vi "Collision Detection top level.vi"(0 "Model rotation (degrees)":sgl, 1 "Model rotation axis (unit vector)":sgl[](array[numeric])=[0.0, 0.0, 1.0], 2 "Traverse Active Parts":cluster{"X":bool, "XY":bool, "XYZ":bool}, 3 "Model rotation axis coordinates (absolute, mm)":sgl[](array[numeric])=[0.0, 0.0, 0.0], 4 "Collision mode":T1=enum."Traverse - All", 5 "Get minimum separation within look-out sphere":bool, 6 "Traverse position (absolute, mm)":sgl[](array[numeric])=[0.0, 0.0, 0.0], 7 "3D graphics output":bool, 9 "Visualisation only (no collision detection)":bool, 10 "Traverse name":string="EnFlo_Trav1", 11 "Extrusion mode":bool, 12 "Rig geometry directory path":path=path "C:/EnFlo_Data_Local/Preferences/Rig_Setups/EnFlo_Tunnel/All_Users/Collision_detection", 13 "Traverse extruded position":sgl[](array[numeric])=[0.0, 0.0, 0.0]) -> (14 "Collision":bool, 15 "Collision point(s)":sgl[][](array[numeric]), 16 "Traverse collision part":cluster{"X":bool, "XY":bool, "XYZ":bool}, 17 "Minimum separation":sgl, 18 "Minimum separation vector (from trav.)":sgl[](array[numeric]), 19 "Error out":errorcluster)   [LabVIEW 2020]
uses:
  Collision Mode.ctl
  Typedefs/Triangle.ctl
  <vilib>/Utility/miscctls.llb/LVRGBAColorTypeDef.ctl
  Convex Hull/Subroutines/Coincident points test.vi
  Subroutines/Cross product 3D.vi
  Subroutines/Unit vector.vi
  Query Octree with triangle.vi
  Tri-Tri intersection test.vi
  Subroutines/Triangle-NodeBox containment test.vi
  Subroutines/Edge-Tri intersection test.vi
  Subroutines/TriVert-in-Box test.vi
  Subroutines/BoxEdges-Tri intersection test.vi
  Subroutines/TriEdges-Box intersection test.vi
  Subroutines/Point-in-Tri test.vi
  Subroutines/Edge-Plane intersection test.vi
  Subroutines/Point-in-Box test (axis-aligned).vi
  Subroutines/Edge-Quad intersection test.vi
  Subroutines/Point-in-Quad test (axis-aligned).vi
  Collision Detection global.vi
  Globals/Trav_pos_global.vi
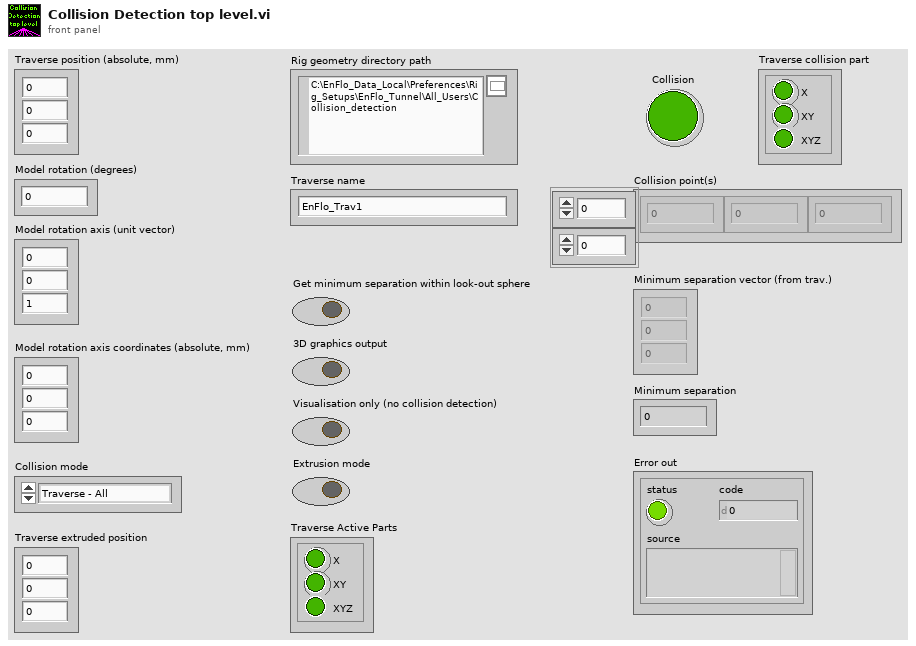
[diagram p1: front panel]
types:
  T1 = typedef "Collision Mode.ctl" = enum16{"Traverse - Tunnel", "Traverse - Model", "Traverse - Fixed objects", "Traverse - Traverse", "Traverse - All"}
  T2 = cluster{"Red":sgl, "Green":sgl, "Blue":sgl, "Alpha":sgl}
  T3 = typedef "LVRGBAColorTypeDef.ctl" = cluster{"Red":sgl, "Green":sgl, "Blue":sgl, "Alpha":sgl}
  T4 = typedef "TreeNodeBox.ctl" = cluster{"Face 0":T5, "Face 1":T5, "Face 2":T5, "Face 3":T5, "Face 4":T5, "Face 5":T5, "Level":i32, "Pmax":sgl[], "Pmin":sgl[], "Parent":i32, "Child 1":i32, "Child 2":i32, "Child 3":i32, "Child 4":i32, "Child 5":i32, "Child 6":i32, "Child 7":i32, "Child 8":i32, "Triangles":i32[], "is leaf node":bool}
  T5 = typedef "Quad.ctl" = cluster{"V0":sgl[], "V1":sgl[], "V2":sgl[], "V3":sgl[], "E0":sgl[], "E1":sgl[], "E2":sgl[], "E3":sgl[], "n^":sgl[], "Plane":T6}
  T6 = typedef "Quadplane enum.ctl" = enum8{"XY", "XZ", "YZ", "-XY", "-XZ", "-YZ"}
  T7 = typedef "Triangle.ctl" = cluster{"V0":sgl[], "V1":sgl[], "V2":sgl[], "E0":sgl[], "E1":sgl[], "E2":sgl[], "n^":sgl[], "nE0^":sgl[], "nE1^":sgl[], "nE2^":sgl[]}
  T8 = typedef "Sphere.ctl" = cluster{"Centre":sgl[], "Radius":sgl}
  T9 = typedef "Triangle, indexed.ctl" = cluster{"V0":sgl[], "V1":sgl[], "V2":sgl[], "n^":sgl[], "i0":i32, "i1":i32, "i2":i32}
  T10 = enum16{"Inherit Value", "Points", "Wireframe", "Polygons"}
  T11 = typedef "LV3DPointTypeDef.ctl" = cluster{"X":sgl, "Y":sgl, "Z":sgl}
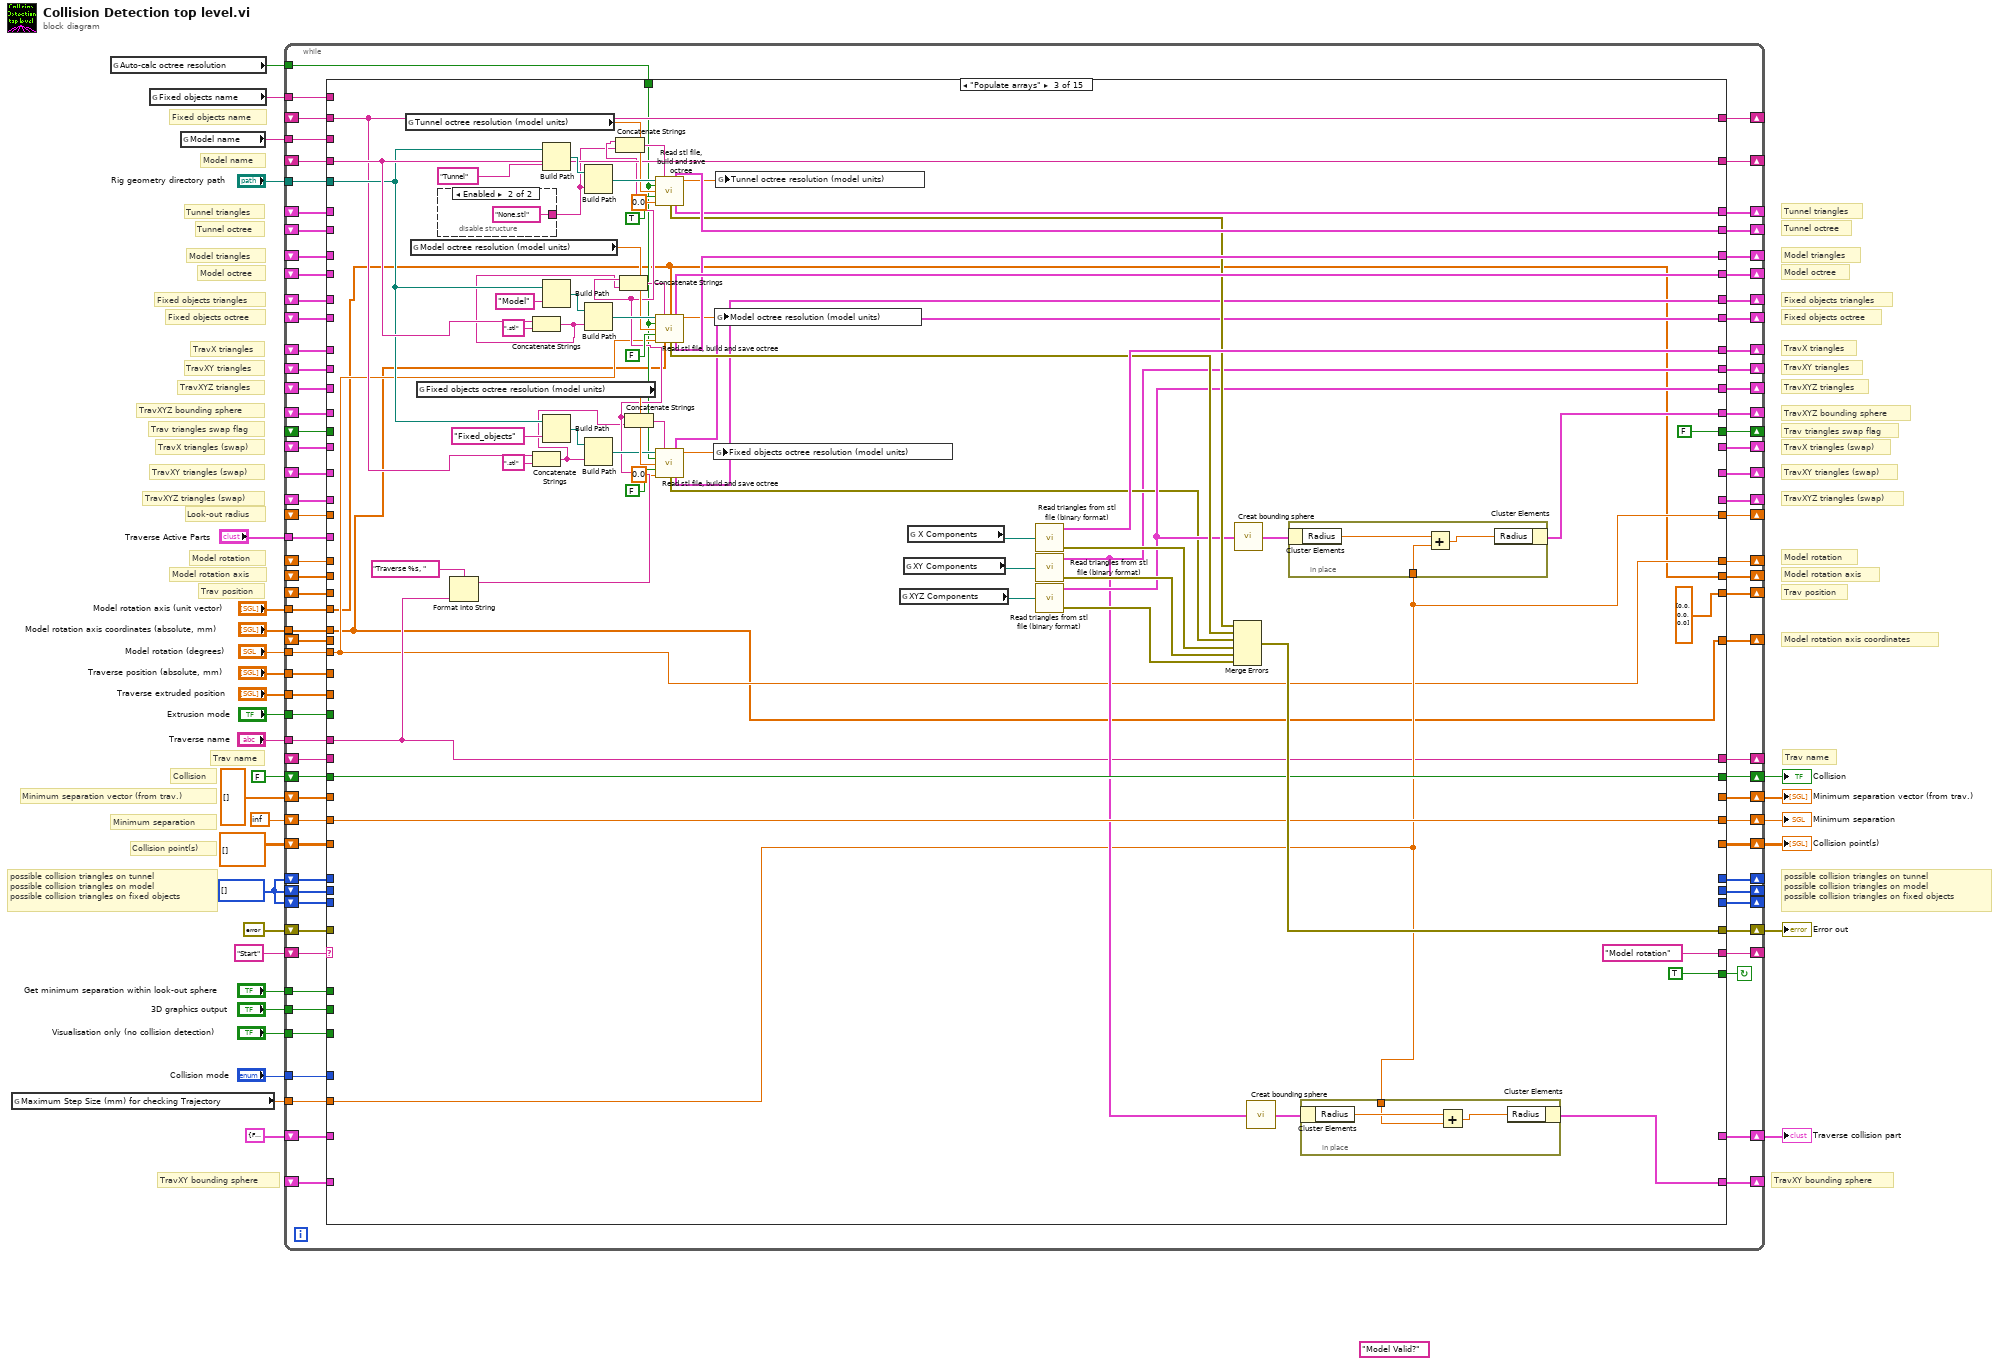
[diagram p0: block diagram]
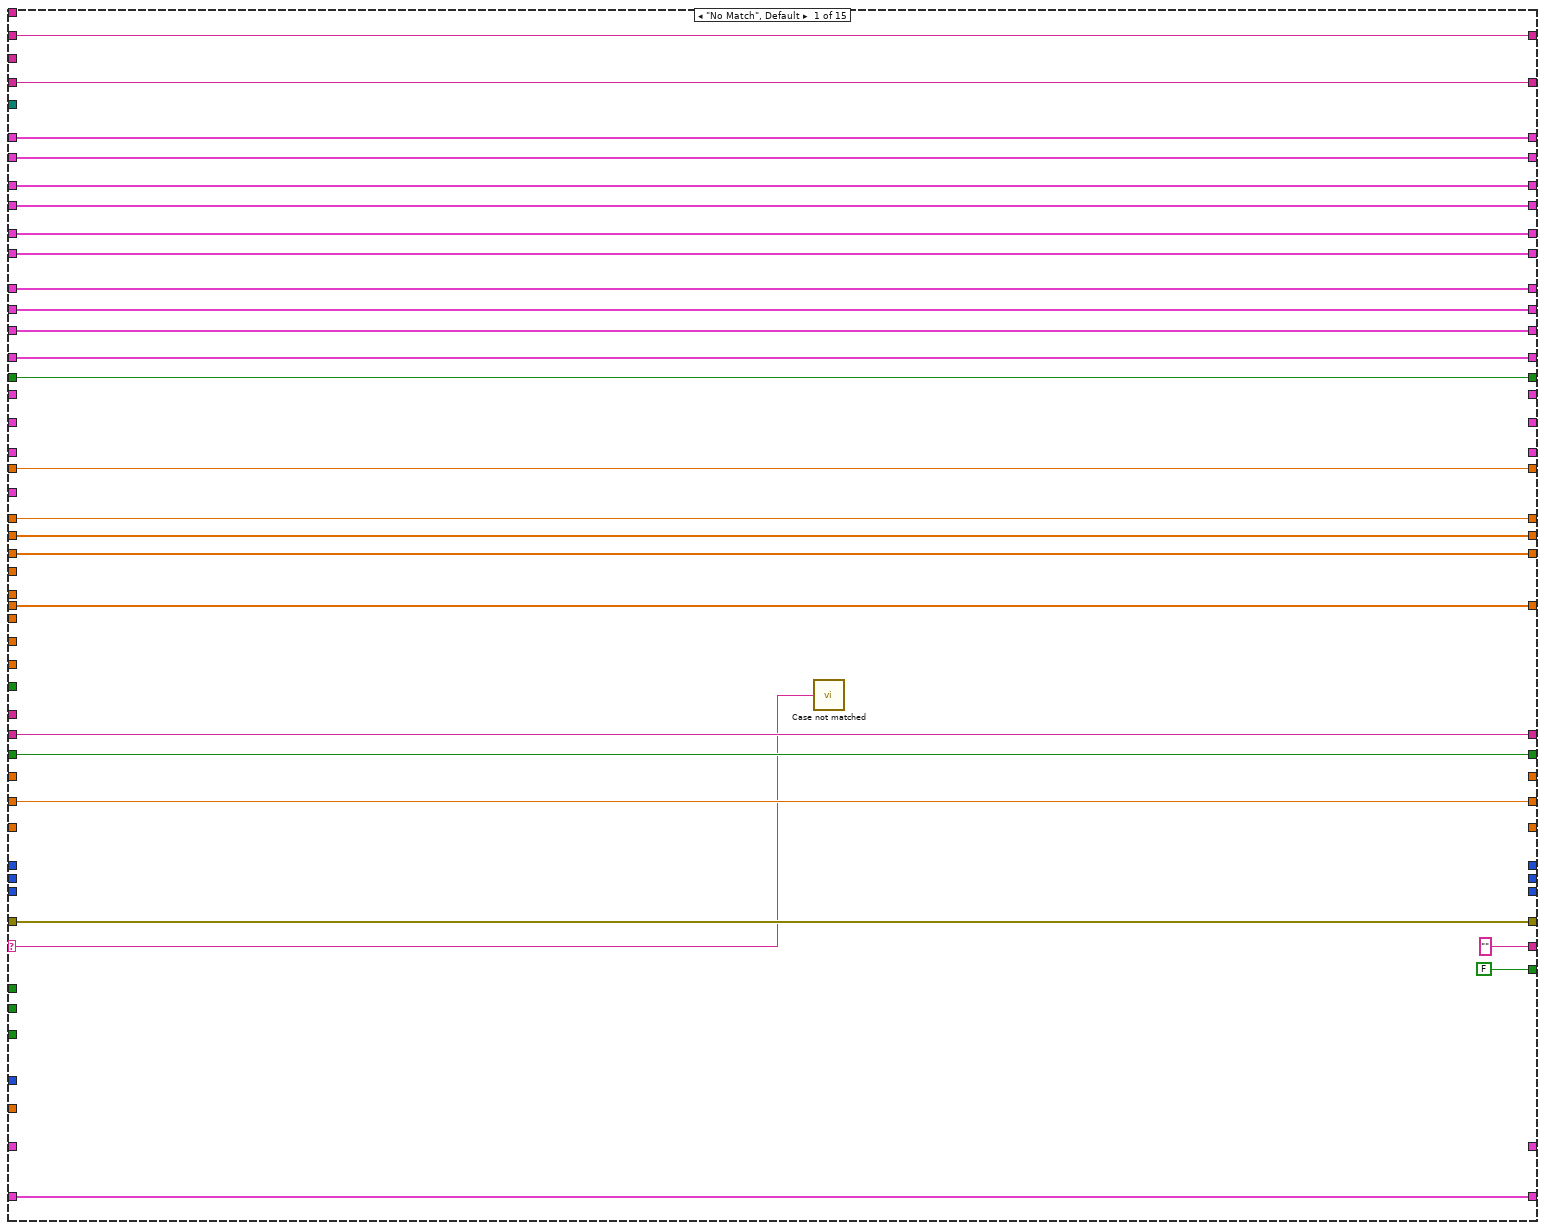
[diagram p2: hidden frame]
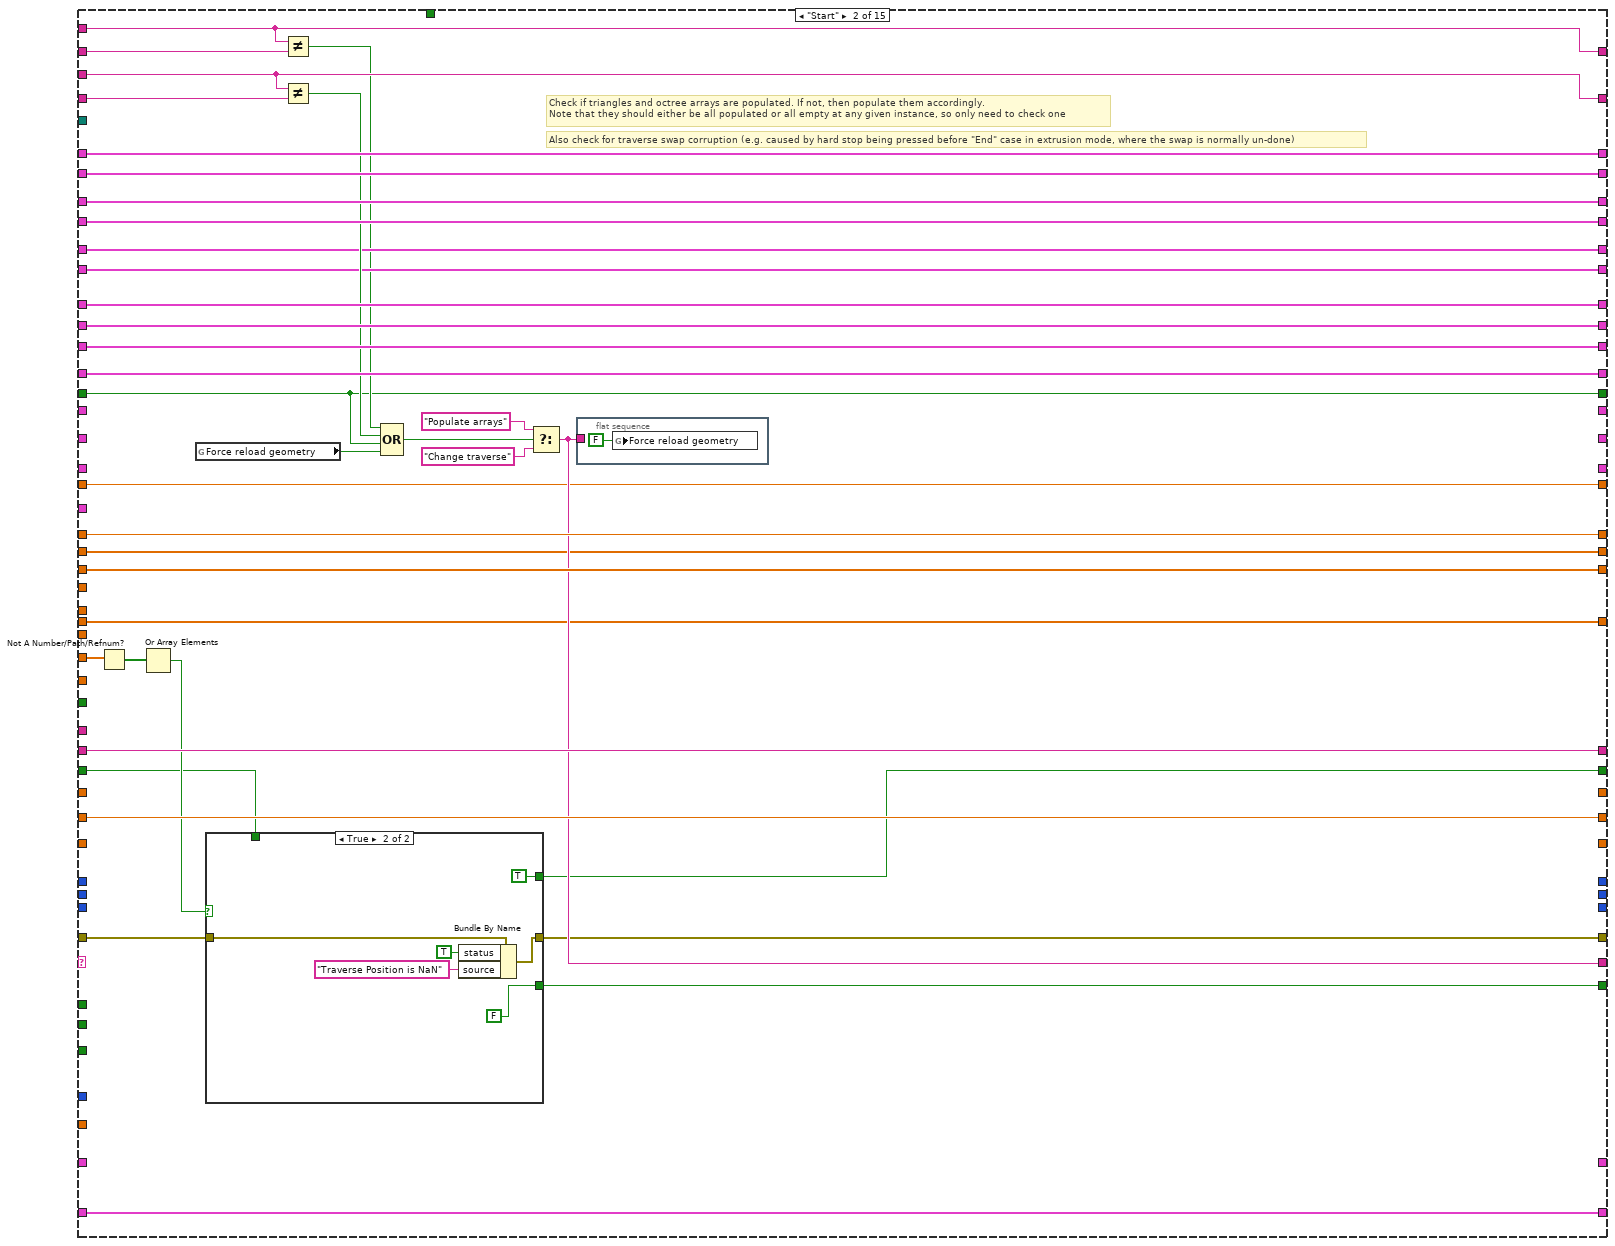
[diagram p3: hidden frame]
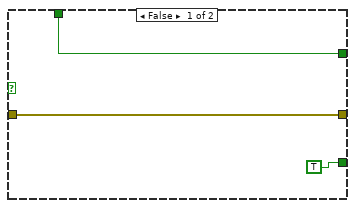
[diagram p4: hidden frame]
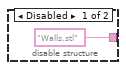
[diagram p5: hidden frame]
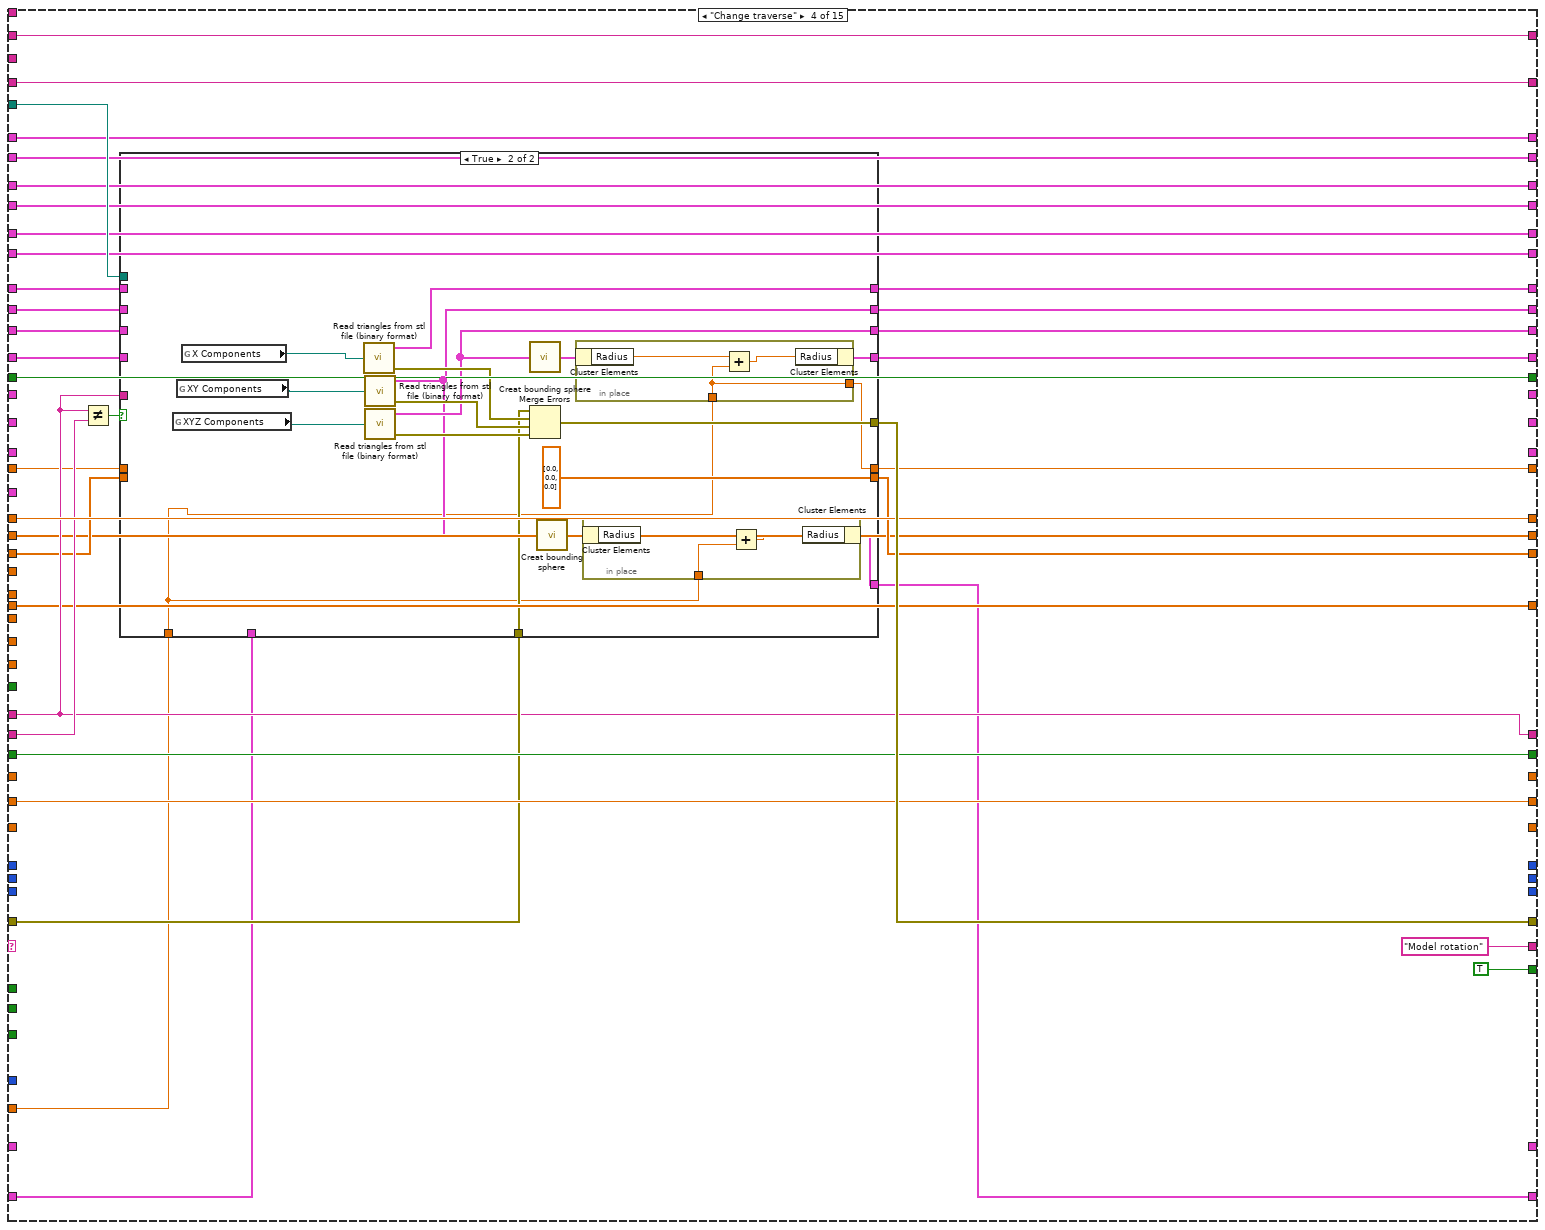
[diagram p6: hidden frame]
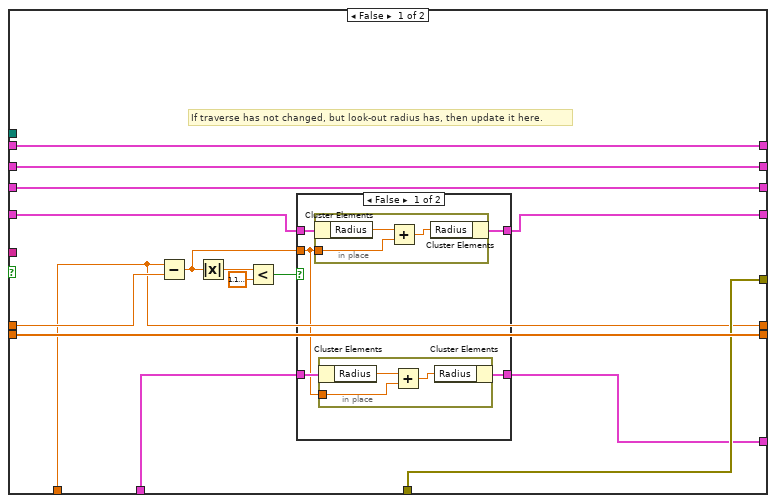
[diagram p7: hidden frame]
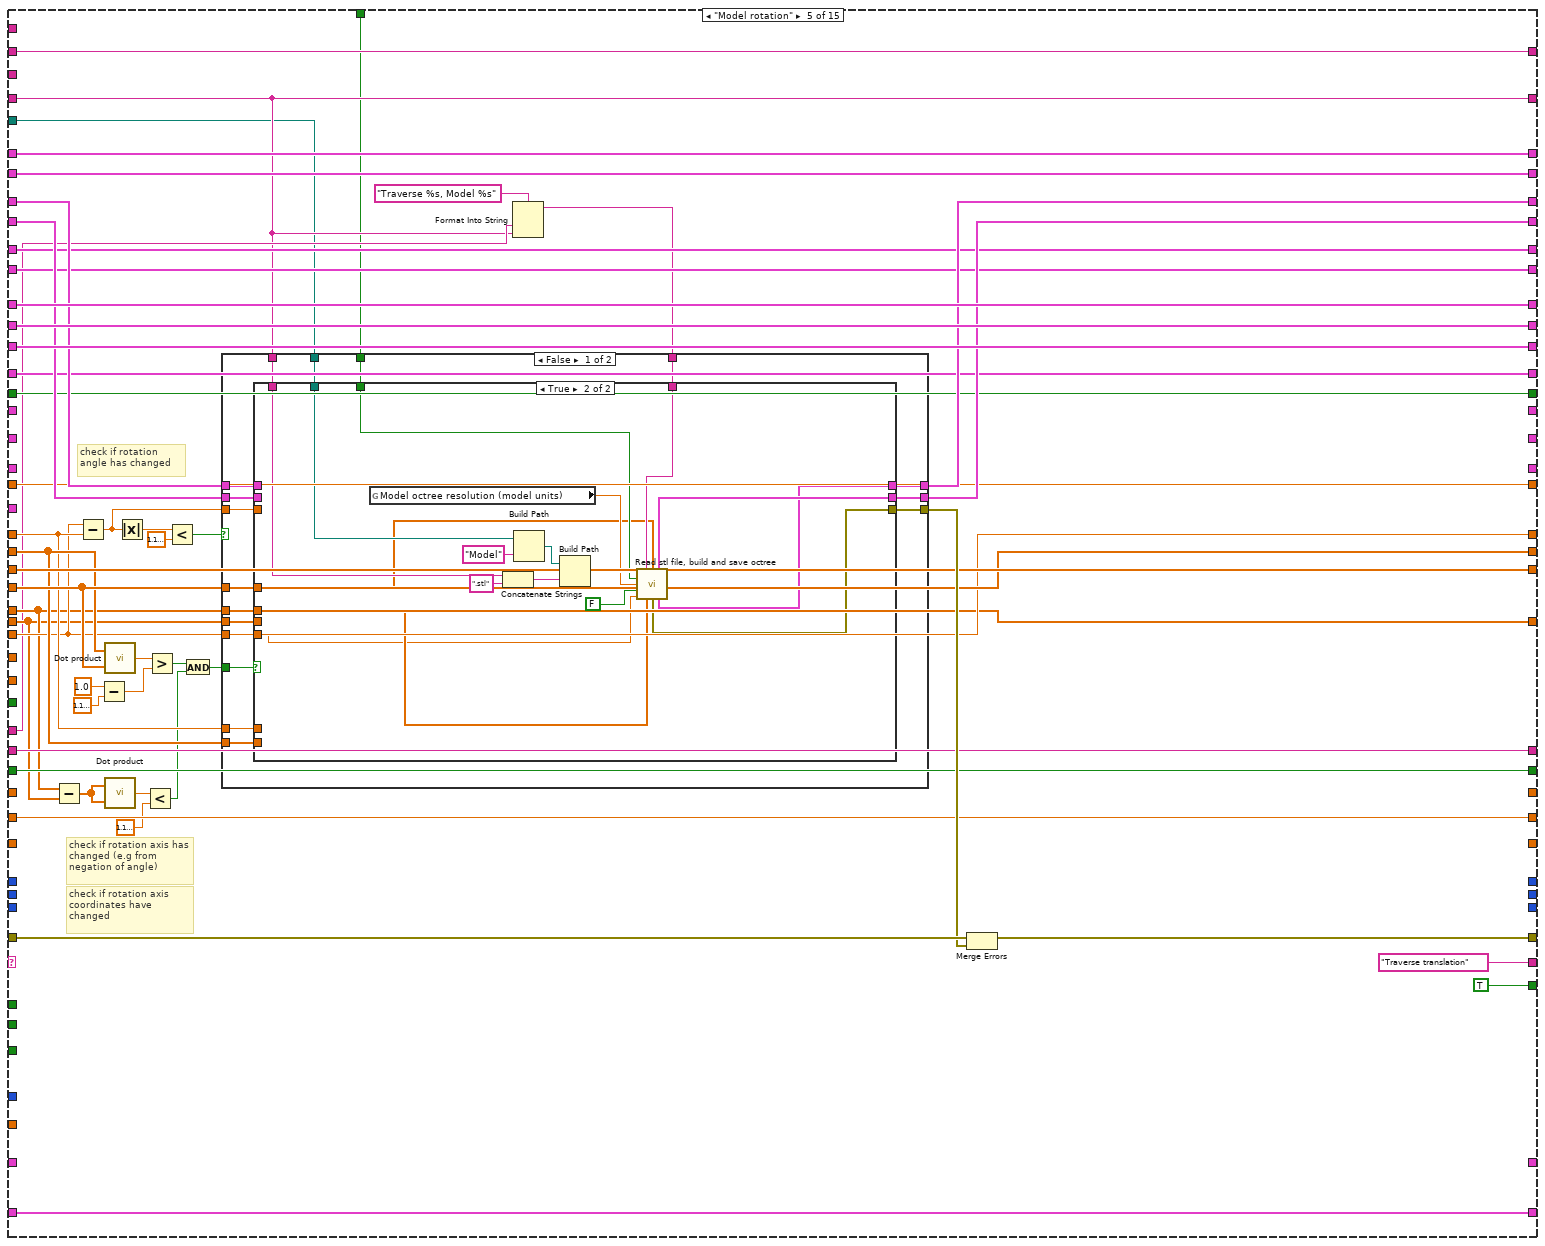
[diagram p9: hidden frame]
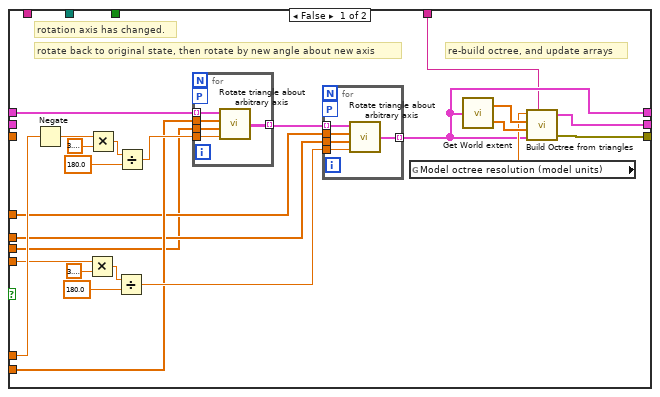
[diagram p10: hidden frame]
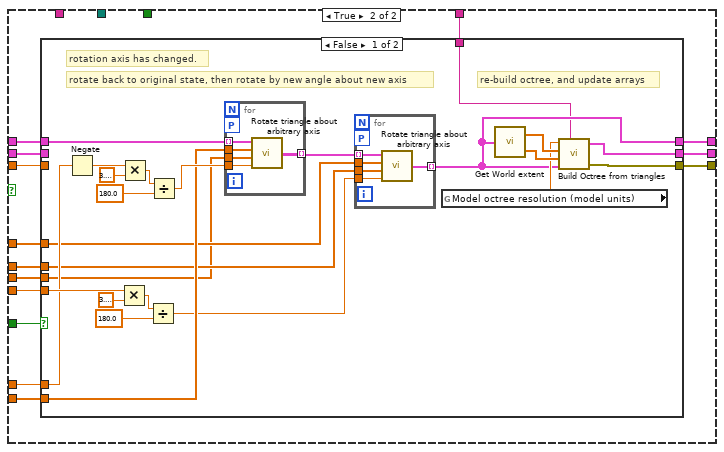
[diagram p11: hidden frame]
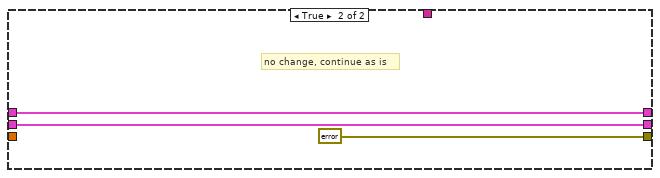
[diagram p12: hidden frame]
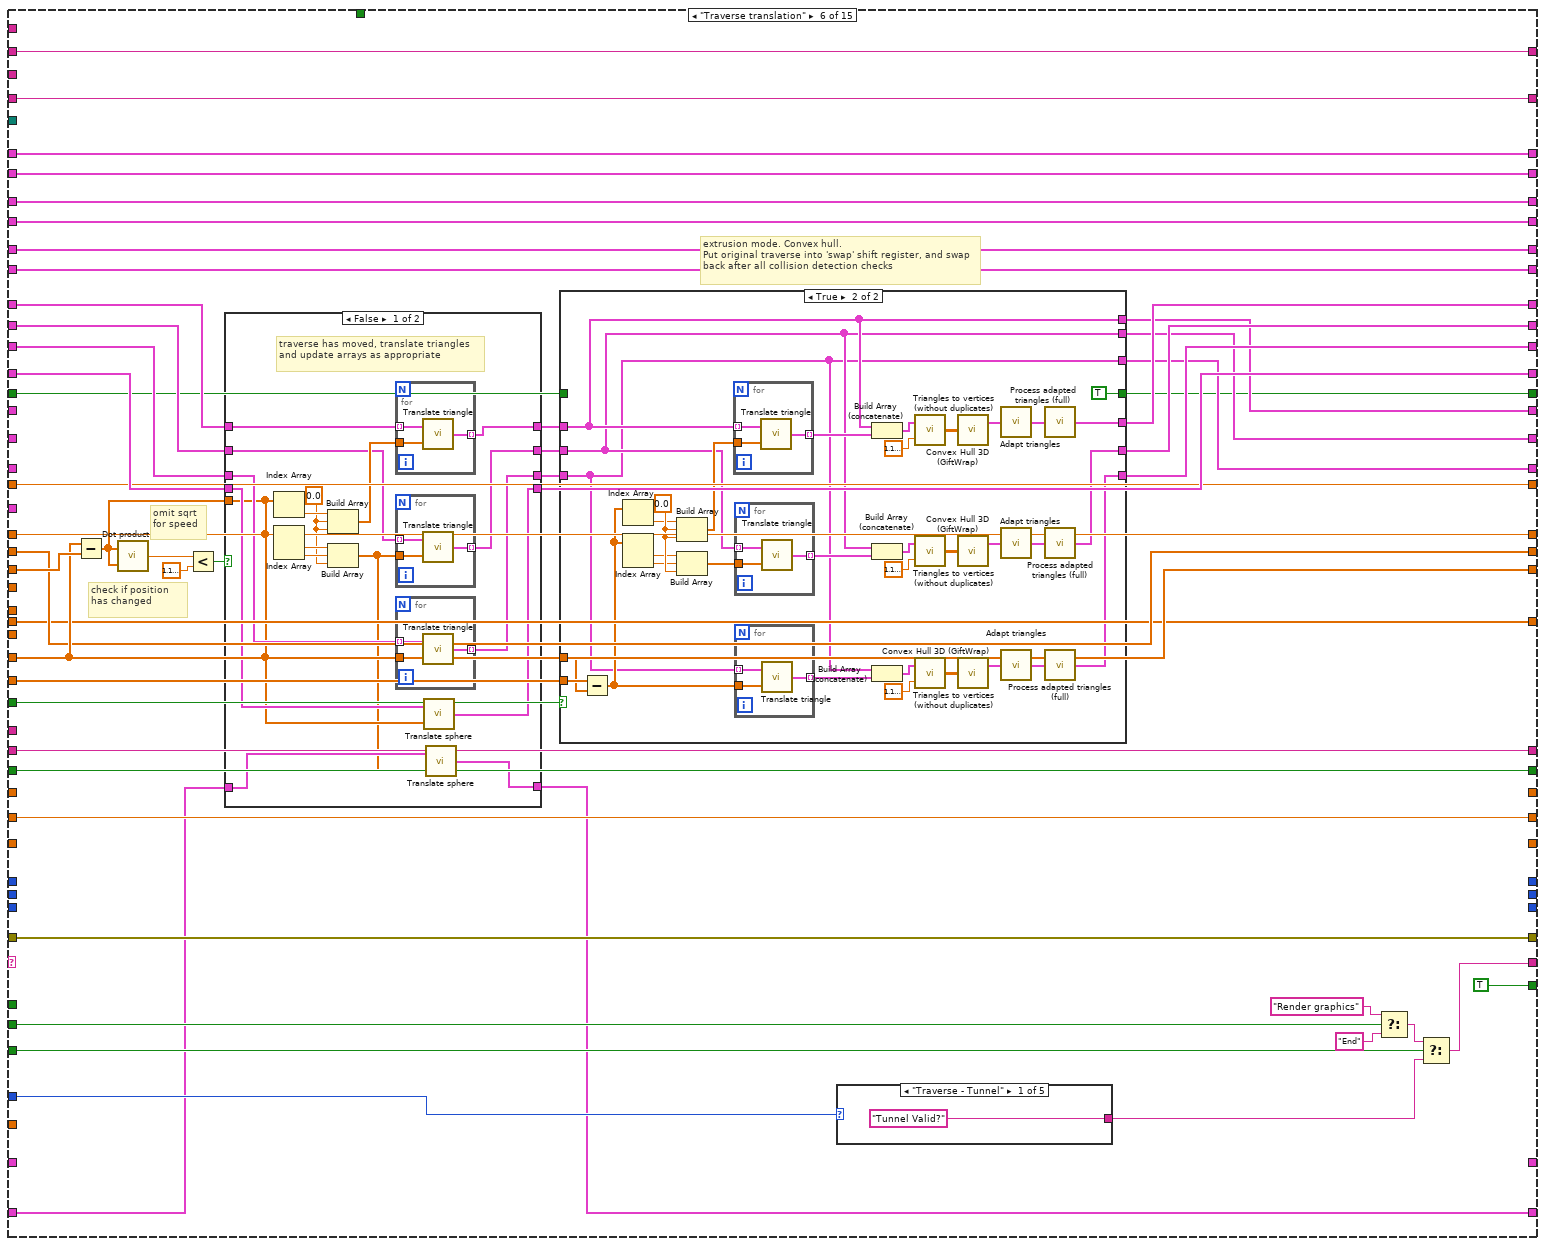
[diagram p13: hidden frame]
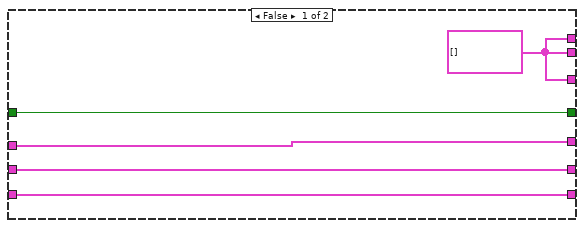
[diagram p14: hidden frame]
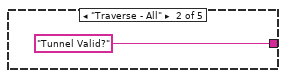
[diagram p15: hidden frame]
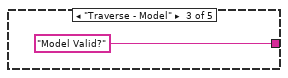
[diagram p16: hidden frame]
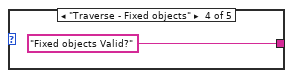
[diagram p17: hidden frame]
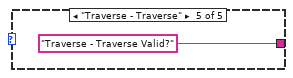
[diagram p18: hidden frame]
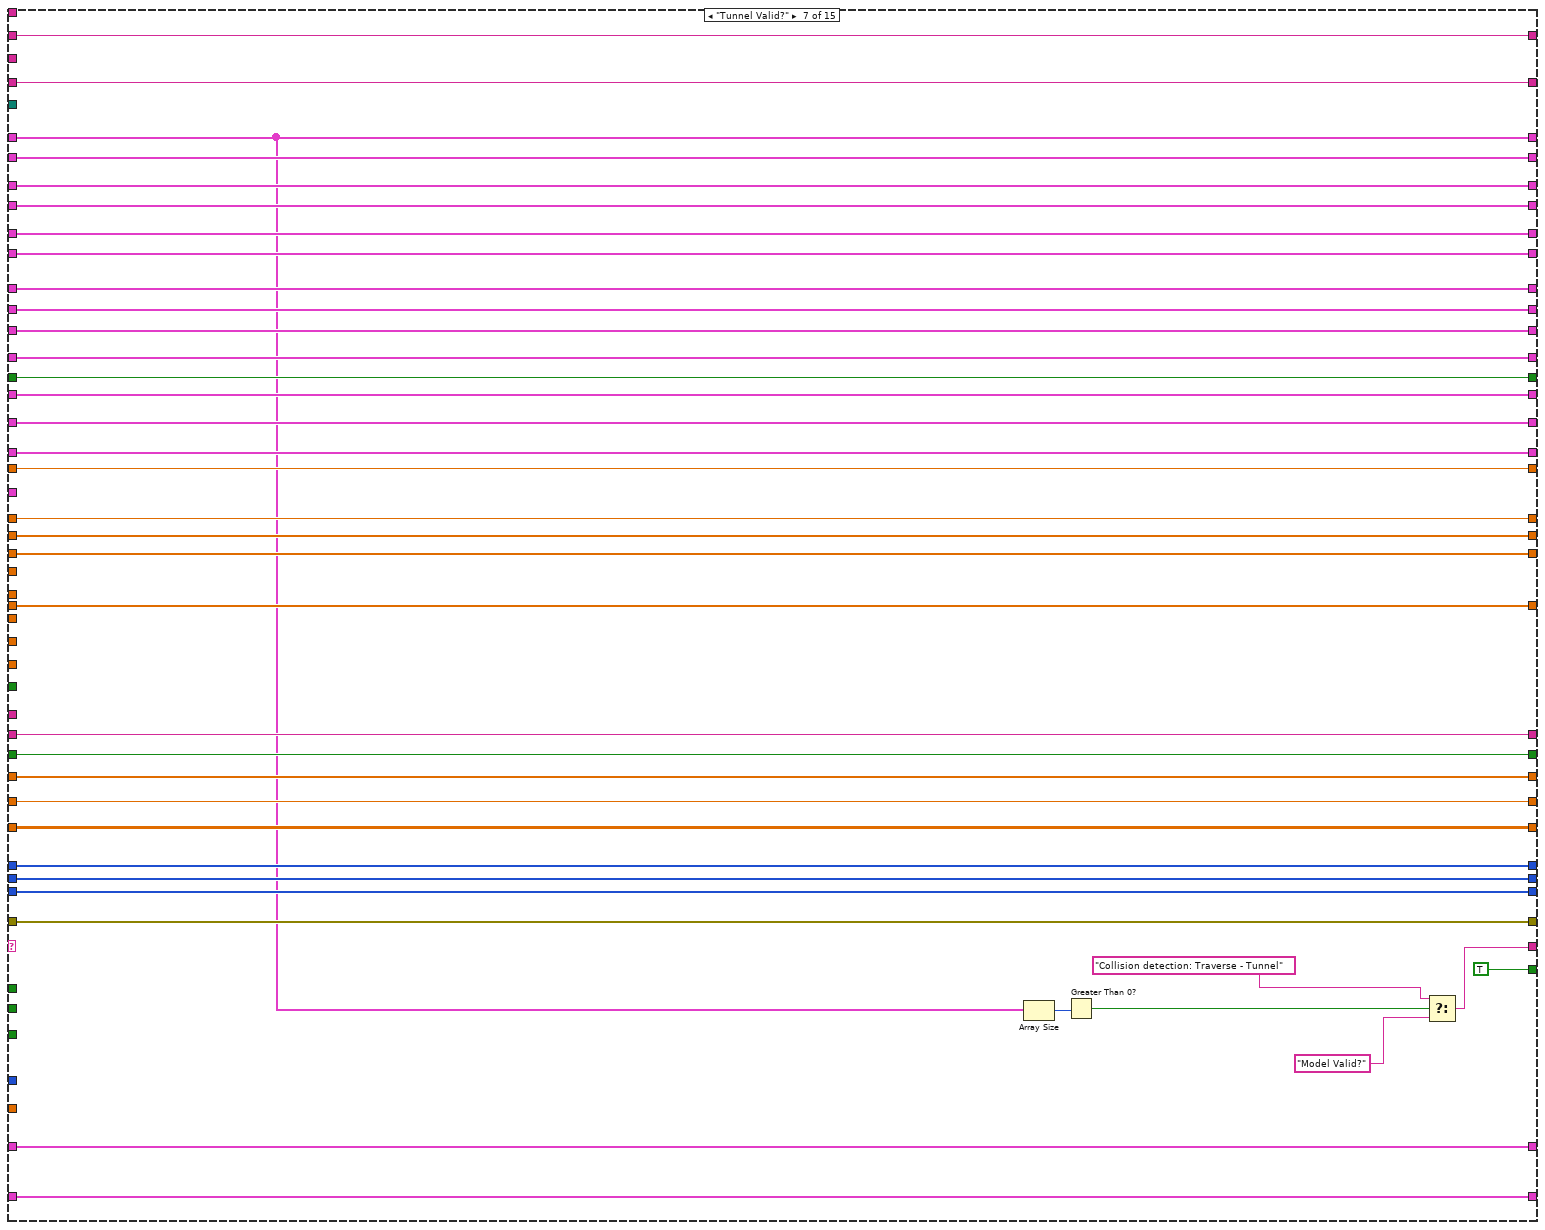
[diagram p20: hidden frame]
diagram:
  (unwired) "Model Valid?"
  w6 = i32[] [] ("I32 array without duplicates")
  # "TravXY bounding sphere"
  # "TravXY bounding sphere"
  # "Look-out radius"
  # "Trav triangles swap flag"
  # "Trav triangles swap flag"
  # "Model rotation axis coordinates"
  # "Model rotation axis"
  # "Model rotation axis"
  # "Fixed objects octree"
  # "Fixed objects triangles"
  # "possible collision triangles on tunnel\npossible collision triangles on model\npossible collision triangles on fixed objects"
  # "Fixed objects name"
  # "Fixed objects octree"
  # "Fixed objects triangles"
  # "Model name"
  # "TravXYZ triangles (swap)"
  # "TravXY triangles (swap)"
  # "TravX triangles (swap)"
  # "TravXYZ triangles (swap)"
  # "TravXY triangles (swap)"
  # "TravX triangles (swap)"
  # "TravXYZ bounding sphere"
  # "TravXYZ bounding sphere"
  # "Trav name"
  # "Collision"
  # "Minimum separation vector (from trav.)"
  # "Minimum separation"
  # "Collision point(s)"
  # "Trav name"
  # "possible collision triangles on tunnel\npossible collision triangles on model\npossible collision triangles on fixed objects"
  # "Model rotation"
  # "Trav position"
  # "TravXYZ triangles"
  # "TravXY triangles"
  # "TravX triangles"
  # "Model octree"
  # "Model triangles"
  # "Tunnel octree"
  # "Tunnel triangles"
  # "Model rotation"
  # "Trav position"
  # "TravXYZ triangles"
  # "TravXY triangles"
  # "TravX triangles"
  # "Model octree"
  # "Model triangles"
  # "Tunnel octree"
  # "Tunnel triangles"
  n1 = global read "Trav_pos_global.vi" "Maximum Step Size (mm) for checking Trajectory"() -> (w2:sgl)
  n2 = global read "Collision Detection global.vi" "Auto-calc octree resolution"() -> (w1:bool)
  n3 = global read "Collision Detection global.vi" "Fixed objects name"() -> (w7:string)
  n4 = global read "Collision Detection global.vi" "Model name"() -> (w9:string)
  n5 = while {
    shift-right: [w97] -> _
    shift-left: "Start" -> [w115]
    shift-right: [w104] -> _
    shift-left: _ -> [w114]
    shift-right: [w103] -> _
    shift-left: _ -> [w113]
    shift-right: [w102] -> _
    shift-left: _ -> [w112]
    shift-right: [w101] -> _
    shift-left: _ -> [w111]
    shift-right: [w100] -> _
    shift-left: _ -> [w110]
    shift-right: [w99] -> _
    shift-left: _ -> [w109]
    shift-right: [w98] -> _
    shift-left: _ -> [w87]
    shift-right: [w91] -> _
    shift-left: _ -> [w107]
    shift-right: [w90] -> _
    shift-left: _ -> [w108]
    tunnel: "Traverse position (absolute, mm)" -> [w105]
    tunnel: "Model rotation (degrees)" -> [w106]
    tunnel: "Rig geometry directory path" -> [w95]
    shift-right: [w93] -> w18
    shift-left: errorcluster {"status"=FALSE, "code"=0, "source"=""} ("error IO") -> [w92]
    tunnel: "Model rotation axis (unit vector)" -> [w89]
    tunnel: "Model rotation axis coordinates (absolute, mm)" -> [w88]
    tunnel: "Get minimum separation within look-out sphere" -> [w86]
    tunnel: "Visualisation only (no collision detection)" -> [w85]
    tunnel: "3D graphics output" -> [w84]
    shift-right: [w80] -> _
    shift-left: w6 -> [w78]
    shift-right: [w79] -> _
    shift-left: w6 -> [w77]
    shift-right: [w81] -> w20
    shift-left: sgl[] [] -> [w76]
    shift-right: [w82] -> w21
    shift-left: sgl inf -> [w75]
    shift-right: [w69] -> w19
    shift-left: sgl[][] [] -> [w74]
    shift-right: [w83] -> w22
    shift-left: FALSE -> [w73]
    shift-right: [w72] -> _
    shift-left: _ -> [w94]
    tunnel: "Traverse name" -> [w71]
    tunnel: "Collision mode" -> [w70]
    shift-right: [w67] -> _
    shift-left: _ -> [w68]
    tunnel: "Traverse extruded position" -> [w66]
    tunnel: "Extrusion mode" -> [w65]
    shift-right: [w64] -> _
    shift-left: _ -> [w61]
    shift-right: [w63] -> _
    shift-left: _ -> [w60]
    shift-right: [w62] -> _
    shift-left: _ -> [w59]
    tunnel: "Traverse Active Parts" -> [w58]
    tunnel: w9 -> [w57]
    shift-right: [w55] -> _
    shift-left: _ -> [w56]
    shift-right: [w52] -> _
    shift-left: _ -> [w54]
    shift-right: [w51] -> _
    shift-left: _ -> [w53]
    tunnel: w7 -> [w50]
    shift-right: [w48] -> _
    shift-left: _ -> [w49]
    shift-right: [w46] -> _
    shift-left: w6 -> [w47]
    shift-right: [w44] -> _
    shift-left: _ -> [w45]
    shift-right: [w42] -> _
    shift-left: _ -> [w43]
    shift-right: [w40] -> w5
    shift-left: cluster{"X":bool, "XY":bool, "XYZ":bool} {"X"=FALSE, "XY"=FALSE, "XYZ"=FALSE} ("Traverse collision part") -> [w41]
    shift-right: [w38] -> _
    shift-left: _ -> [w39]
    shift-right: [w36] -> _
    shift-left: _ -> [w37]
    shift-right: [w35] -> _
    shift-left: _ -> [w34]
    tunnel: w2 -> [w33]
    tunnel: w1 -> [w32]
    stop <- w96 continue-if-true
    n6 = case shown="\"Populate arrays\"" w115 {
      selector: w115 -> [w116 _ _ _ _ _ _ _ _ _ _ _ _ _ _]
      tunnel: w114 -> [w138 w171 _ w292 w403 w568 w663 w721 w830 w926 w1067 w1163 w1326 w1410 w1567]
      tunnel: w113 -> [w137 w172 _ w291 w402 w567 w691 w722 w857 w925 w1093 w1162 w1325 w1406 w1566]
      tunnel: w112 -> [w136 w164 _ w290 w398 w566 w688 w742 w827 w865 w1064 w1143 w1322 w1368 w1565]
      tunnel: w111 -> [w135 w173 _ w289 w393 w565 w687 w741 w854 w878 w1090 w1142 w1321 w1405 w1564]
      tunnel: w110 -> [w134 w174 _ w285 w401 w572 w692 w744 w858 w927 w1094 w1164 w1327 w1409 w1551]
      tunnel: w109 -> [w133 w175 _ w284 w400 w571 w690 w743 w856 w873 w1092 w1111 w1324 w1408 w1552]
      tunnel: w87 -> [w132 w176 _ w283 w399 w570 w689 w723 w855 w877 w1091 w1115 w1323 w1407 w1553]
      tunnel: w108 -> [w130 w169 _ w281 w385 w575 w696 w747 w862 w930 w1098 w1167 w1334 w1414 w1569]
      tunnel: w107 -> [w131 w170 _ w295 w374 w552 w697 w748 w863 w931 w1099 w1168 w1335 w1415 w1568]
      tunnel: w106 -> [_ _ w193 _ w373 _ _ _ _ _ _ _ _ _ _]
      tunnel: w105 -> [_ w149 _ _ _ w545 _ _ _ _ _ _ _ _ _]
      tunnel: [w138 w171 w253 w292 w403 w568 w663 w721 w830 w926 w1067 w1163 w1326 w1410 w1567] -> w104
      tunnel: [w137 w172 w254 w291 w402 w567 w691 w722 w857 w925 w1093 w1162 w1325 w1406 w1566] -> w103
      tunnel: [w136 w164 w255 w290 w395 w566 w688 w742 w827 w865 w1064 w1143 w1322 w1368 w1565] -> w102
      tunnel: [w135 w173 w256 w289 w394 w565 w687 w741 w854 w878 w1090 w1142 w1321 w1405 w1564] -> w101
      tunnel: [w134 w174 w257 w300 w401 w541 w692 w744 w858 w927 w1094 w1164 w1327 w1409 w1556] -> w100
      tunnel: [w133 w175 w210 w301 w400 w540 w690 w743 w856 w873 w1092 w1111 w1324 w1408 w1555] -> w99
      tunnel: [w132 w176 w233 w302 w399 w539 w689 w723 w855 w877 w1091 w1115 w1323 w1407 w1554] -> w98
      tunnel: [w131 w170 w193 w295 w373 w552 w697 w748 w863 w931 w1099 w1168 w1335 w1415 w1568] -> w91
      tunnel: [w130 w169 sgl[] [0.0, 0.0, 0.0] ("Traverse position (absolute, mm)") w280 w385 w545 w696 w747 w862 w930 w1098 w1167 w1334 w1414 w1569] -> w90
      tunnel: w95 -> [_ _ w221 w299 w356 _ _ _ _ _ _ _ _ _ _]
      tunnel: ["" w166 "Model rotation" "Model rotation" "Traverse translation" w561 w694 "Model Valid?" w860 "Fixed objects Valid?" w1096 "Collision detection: Traverse - Traverse" w1330 "End" "" ("f")] -> w97
      tunnel: [FALSE w144 TRUE TRUE TRUE TRUE TRUE TRUE TRUE TRUE TRUE TRUE TRUE TRUE FALSE] -> w96
      tunnel: w94 -> [w127 w167 _ w287 w386 w554 w686 w738 w853 w924 w1089 w1161 w1320 w1375 w1562]
      tunnel: [w139 w146 w252 w298 w392 w563 w693 w745 w859 w928 w1095 w1165 w1328 w1393 w1570] -> w93
      tunnel: w92 -> [w139 w145 _ w288 w391 w563 w693 w745 w859 w928 w1095 w1165 w1328 w1394 w1570]
      tunnel: w89 -> [_ _ w191 _ w380 _ _ _ _ _ _ _ _ _ _]
      tunnel: w88 -> [_ _ w190 _ w367 _ _ _ _ _ _ _ _ _ _]
      tunnel: w86 -> [_ _ _ _ _ _ _ w727 _ w906 _ w1141 _ _ w1537]
      tunnel: w85 -> [_ _ _ _ _ w562 _ _ _ _ _ _ _ _ _]
      tunnel: w84 -> [_ _ _ _ _ w560 _ _ _ _ _ _ w1331 _ _]
      tunnel: [w128 w143 w236 w293 w387 w555 w685 w728 w852 w907 w1088 w1144 w1319 w1411 w1563] -> w83
      tunnel: [w129 w168 w237 w294 w388 w556 w683 w740 w850 w920 w1086 w1157 w1317 w1412 w1538] -> w82
      tunnel: [_ _ _ _ _ _ w684 w739 w851 w919 w1087 w1156 w1318 w1413 w1540] -> w81
      tunnel: [_ _ _ _ _ _ w680 w737 w847 w922 w1083 w1159 w1314 w1343 w1546] -> w69
      tunnel: [_ _ _ _ _ _ w682 w724 w849 w923 w1085 w1160 w1316 _ _] -> w80
      tunnel: [_ _ _ _ _ _ w681 _ w848 _ w1084 w1106 w1315 _ _] -> w79
      tunnel: w78 -> [_ _ _ _ _ _ w682 _ w849 w923 w1085 w1160 w1316 w1385 _]
      tunnel: w77 -> [_ _ _ _ _ _ w681 _ w848 _ w1084 _ w1315 w1344 _]
      tunnel: w76 -> [_ _ _ _ _ _ w684 _ w851 w874 w1087 w1104 w1318 w1413 w1540]
      tunnel: w75 -> [w129 w168 w237 w294 w388 w556 w683 _ w850 w875 w1086 w1103 w1317 w1412 w1539]
      tunnel: w74 -> [_ _ _ _ _ _ w680 _ w847 w902 w1083 w1137 w1314 w1343 w1546]
      tunnel: w73 -> [w128 w142 w236 w293 w387 w555 w685 _ w852 w916 w1088 w1153 w1319 w1411 w1563]
      tunnel: [w127 w167 w206 w282 w386 w554 w686 w738 w853 w924 w1089 w1161 w1320 w1375 w1562] -> w72
      tunnel: w71 -> [_ _ w206 w282 w359 _ _ _ _ _ _ _ _ _ _]
      tunnel: w70 -> [_ _ _ _ _ w551 _ _ _ _ _ _ _ _ _]
      tunnel: w68 -> [w126 w165 _ w278 w384 w549 w679 w720 w846 w879 w1082 w1112 w1313 w1362 w1561]
      tunnel: [w126 w165 w231 w279 w384 w548 w679 w720 w846 w879 w1082 w1112 w1313 w1362 w1561] -> w67
      tunnel: w66 -> [_ _ _ _ _ w546 _ _ _ _ _ _ _ _ _]
      tunnel: w65 -> [_ _ _ _ _ w547 _ _ _ _ _ _ _ _ w1560]
      tunnel: [_ _ _ _ _ w536 w678 w719 w845 w905 w1081 w1140 w1312 w1361 _] -> w64
      tunnel: [_ _ _ _ _ w537 w677 w718 w844 w904 w1080 w1139 w1311 w1360 _] -> w63
      tunnel: [_ _ _ _ _ w538 w676 w717 w843 w903 w1079 w1138 w1310 w1359 _] -> w62
      tunnel: w61 -> [_ _ _ _ _ _ w678 w719 w845 w905 w1081 w1140 w1312 w1361 w1559]
      tunnel: w60 -> [_ _ _ _ _ _ w677 w718 w844 w904 w1080 w1139 w1311 w1360 w1558]
      tunnel: w59 -> [_ _ _ _ _ _ w676 w717 w843 w903 w1079 w1138 w1310 w1359 w1557]
      tunnel: w58 -> [_ _ _ _ _ _ _ w701 _ w881 _ w1117 _ _ _]
      tunnel: w57 -> [_ w163 _ _ _ _ _ _ _ _ _ _ _ _ _]
      tunnel: w56 -> [w125 w162 w228 w277 w357 w535 w675 w715 w842 w900 w1078 w1135 w1309 w1357 w1550]
      tunnel: [w125 w163 w228 w277 w357 w535 w675 w715 w842 w900 w1078 w1135 w1309 w1357 w1550] -> w55
      tunnel: w54 -> [w124 w160 _ w275 w381 w533 w673 w713 w840 w898 w1063 w1114 w1307 w1352 w1548]
      tunnel: w53 -> [w123 w159 _ w274 w382 w532 w672 w712 w839 w897 w1076 w1113 w1306 w1355 w1547]
      tunnel: [w124 w160 w218 w275 w381 w533 w673 w713 w840 w898 w1063 w1114 w1307 w1352 w1548] -> w52
      tunnel: [w123 w159 w217 w274 w382 w532 w672 w712 w839 w897 w1076 w1113 w1306 w1355 w1547] -> w51
      tunnel: w50 -> [_ w156 _ _ _ _ _ _ _ _ _ _ _ _ _]
      tunnel: w49 -> [w122 w158 w220 w276 w383 w534 w674 w714 w841 w899 w1077 w1134 w1308 w1356 w1549]
      tunnel: [w122 w156 w220 w276 w383 w534 w674 w714 w841 w899 w1077 w1134 w1308 w1356 w1549] -> w48
      tunnel: w47 -> [_ _ _ _ _ _ w671 _ w838 _ w1075 w1133 w1305 w1345 _]
      tunnel: [_ _ _ _ _ _ w671 _ w838 w867 w1075 w1133 w1305 _ _] -> w46
      tunnel: w45 -> [w121 w155 _ w273 w375 w531 w670 w711 w837 w896 w1074 w1132 w1304 w1342 w1545]
      tunnel: [w121 w155 w191 w273 w380 w531 w670 w711 w837 w896 w1074 w1132 w1304 w1342 w1545] -> w44
      tunnel: w43 -> [w120 w154 _ w272 w364 w530 w669 w710 w836 w895 w1073 w1131 w1303 w1341 w1544]
      tunnel: [w120 w154 w190 w272 w367 w530 w669 w710 w836 w895 w1073 w1131 w1303 w1341 w1544] -> w42
      tunnel: w41 -> [_ _ _ _ _ _ w668 _ w835 w894 w1072 w1124 w1302 w1340 w1543]
      tunnel: [_ _ _ _ _ _ w668 w707 w835 w885 w1072 w1123 w1302 w1340 w1543] -> w40
      tunnel: w39 -> [w119 w152 _ w271 w363 w528 w667 w705 w834 w884 w1071 w1120 w1301 w1339 w1541]
      tunnel: [w119 w152 FALSE w271 w363 w529 w667 w705 w834 w884 w1071 w1120 w1301 w1339 w1542] -> w38
      tunnel: w37 -> [w118 w151 _ w270 w362 w527 w666 w704 w833 w883 w1070 w1119 w1300 w1338 w1536]
      tunnel: [w118 w151 w208 w269 w362 w527 w666 w704 w833 w883 w1070 w1119 w1300 w1338 w1536] -> w36
      tunnel: [w117 w150 w209 w268 w361 w525 w665 w702 w832 w872 w1069 w1110 w1299 w1336 w1535] -> w35
      tunnel: w34 -> [w117 w150 _ w267 w361 w526 w665 w702 w832 w872 w1069 w1110 w1299 w1336 w1535]
      tunnel: w33 -> [_ _ w208 w266 _ _ _ _ _ _ _ _ _ _ _]
      tunnel: w32 -> [_ _ w192 _ w355 _ _ _ _ _ _ _ _ _ _]
      frame "No Match", Default {
        n7 = call "Case not matched.vi"("Case Name not Matched"=w116) -> ()
      }
      frame "Start" {
        # "Also check for traverse swap corruption (e.g. caused by hard stop being pressed before \"End\" case in extrusion mode, where the swap is normally un-done)"
        # "Check if triangles and octree arrays are populated. If not, then populate them accordingly.\nNote that they should either be all populated or all empty at any given instance, so only need to check one"
        n8 = Not A Number/Path/Refnum?(number/path/refnum=w149) -> (NaN/Path/Refnum?=w148:bool[])
        n9 = Or Array Elements(Boolean array=w148) -> (logical OR=w147:bool)
        n10 = global read "Collision Detection global.vi" "Force reload geometry"() -> (w153:bool)
        n11 = case shown="True" w147 {
          tunnel: [w182 w185] -> w146
          tunnel: w145 -> [w182 w188]
          tunnel: [TRUE FALSE] -> w144
          tunnel: [w180 TRUE] -> w143
          tunnel: w142 -> [w180 _]
          frame False {
          }
          frame True {
            n12 = Bundle By Name(cluster=w188, "status"=TRUE, "source"="Traverse Position is NaN") -> (w185:errorcluster)
          }
        }
        n13 = Not Equal?(x=w156, y=w158) -> (x != y?=w157:bool)
        n14 = Not Equal?(x=w163, y=w162) -> (x != y?=w161:bool)
        n15 = Compound Arithmetic op=OR(w157, w161, w152, w153) -> (w179:bool)
        n16 = Select(t="Populate arrays", s=w179, f="Change traverse") -> (s? t:f=w166:string)
        n17 = flat-sequence {
          tunnel: w166 -> [_]
          frame #0 {
            n18 = global write "Collision Detection global.vi" "Force reload geometry"(FALSE ("Force reload geometry")) -> ()
          }
        }
      }
      frame "Populate arrays" {
        n19 = global read "Collision Detection global.vi" "Tunnel octree resolution (model units)"() -> (w235:sgl)
        n20 = global read "Collision Detection global.vi" "Model octree resolution (model units)"() -> (w234:sgl)
        n21 = global read "Collision Detection global.vi" "Fixed objects octree resolution (model units)"() -> (w226:sgl)
        n22 = disable-structure shown="Enabled" {
          disable-tunnel: ["Walls.stl" "None.stl"] -> w198
          frame Disabled {
          }
          frame Enabled {
          }
        }
        n23 = Format Into String(format string="Traverse %s, ", w206) -> (resulting string=w201:string)  [unwired: 2 in, 1 out]
        n24 = Concatenate Strings(w228, ".stl" ("string")) -> (w197:string)
        n25 = Concatenate Strings(w220, ".stl" ("string")) -> (w196:string)
        n26 = Build Path(base path=w221, name or relative path="Tunnel") -> (appended path=w250:path)
        n27 = Build Path(base path=w221, name or relative path="Model") -> (appended path=w247:path)
        n28 = Build Path(base path=w221, name or relative path="Fixed_objects") -> (appended path=w223:path)
        n29 = Build Path(base path=w250, name or relative path=w198) -> (appended path=w251:path)
        n30 = Build Path(base path=w247, name or relative path=w197) -> (appended path=w245:path)
        n31 = Build Path(base path=w223, name or relative path=w196) -> (appended path=w225:path)
        n32 = Concatenate Strings(w201, w198) -> (w200:string)
        n33 = Concatenate Strings(w201, w197) -> (w199:string)
        n34 = Concatenate Strings(w201, w196) -> (w204:string)
        n35 = call "Read stl file, build and save octree.vi"("STL file path (load)"=w251, "String"=w200, "Auto resolution"=w192, "Specify resolution"=w235, "Invert model (interior region)"=TRUE, "Model Rotation (deg)"=sgl 0.0) -> ("Octree node array"=w254:T4[], "Octree resolution"=w230:sgl, "Error out"=w244:errorcluster, "Triangles array"=w253:T7[])  [unwired: 6 in]
        n36 = call "Read stl file, build and save octree.vi"("STL file path (load)"=w245, "String"=w199, "Model rotation axis (unit vector)"=w191, "Auto resolution"=w192, "Specify resolution"=w234, "Invert model (interior region)"=FALSE, "Model Rotation (deg)"=w193, "Model rotation axis coordinates (absolute, mm)"=w190) -> ("Octree node array"=w256:T4[], "Octree resolution"=w229:sgl, "Error out"=w243:errorcluster, "Triangles array"=w255:T7[])  [unwired: 4 in]
        n37 = call "Read stl file, build and save octree.vi"("STL file path (load)"=w225, "String"=w204, "Auto resolution"=w192, "Specify resolution"=w226, "Invert model (interior region)"=FALSE, "Model Rotation (deg)"=sgl 0.0) -> ("Octree node array"=w217:T4[], "Octree resolution"=w227:sgl, "Error out"=w219:errorcluster, "Triangles array"=w218:T7[])  [unwired: 6 in]
        n38 = global write "Collision Detection global.vi" "Fixed objects octree resolution (model units)"(w227) -> ()
        n39 = global write "Collision Detection global.vi" "Model octree resolution (model units)"(w229) -> ()
        n40 = global write "Collision Detection global.vi" "Tunnel octree resolution (model units)"(w230) -> ()
        n41 = global read "Collision Detection global.vi" "XYZ Components"() -> (w212:path)
        n42 = global read "Collision Detection global.vi" "XY Components"() -> (w213:path)
        n43 = global read "Collision Detection global.vi" "X Components"() -> (w214:path)
        n44 = call "Read triangles from stl file (binary format).vi"("STL file path"=w214) -> ("Triangles array"=w257:T7[], "Error out"=w242:errorcluster)  [unwired: 1 out]
        n45 = call "Read triangles from stl file (binary format).vi"("STL file path"=w213) -> ("Triangles array"=w210:T7[], "Error out"=w241:errorcluster)  [unwired: 1 out]
        n46 = call "Read triangles from stl file (binary format).vi"("STL file path"=w212) -> ("Triangles array"=w233:T7[], "Error out"=w240:errorcluster)  [unwired: 1 out]
        n47 = Merge Errors(w244, w243, w219, w242, w241, w240) -> (w252:errorcluster)
        n48 = call "Creat bounding sphere.vi"("Triangles"=w233) -> ("Bounding sphere"=w232:T8)
        n49 = call "Creat bounding sphere.vi"("Triangles"=w210) -> ("Bounding sphere"=w211:T8)
        n50 = in-place {
          in-place-border: w208 -> [w263]
          n51 = in-place-cluster #1(w232) -> ("Radius"=w265:sgl)
          n52 = Add(x=w265, y=w263) -> (x+y=w264:sgl)
          n53 = in-place-cluster #1("Radius"=w264) -> (w231:T8)
        }
        n54 = in-place {
          in-place-border: w208 -> [w260]
          n55 = in-place-cluster #2(w211) -> ("Radius"=w262:sgl)
          n56 = Add(x=w262, y=w260) -> (x+y=w261:sgl)
          n57 = in-place-cluster #2("Radius"=w261) -> (w209:T8)
        }
      }
      frame "Change traverse" {
        n58 = Not Equal?(x=w282, y=w287) -> (x != y?=w286:bool)
        n59 = case shown="True" w286 {
          tunnel: [w315 w341] -> w302
          tunnel: [w316 w333] -> w301
          tunnel: [w317 w348] -> w300
          tunnel: w299 -> [_ _]
          tunnel: [w310 w347] -> w298
          tunnel: w282 -> [_ _]
          tunnel: w288 -> [w310 w343]
          tunnel: w285 -> [w317 _]
          tunnel: w284 -> [w316 _]
          tunnel: w283 -> [w315 _]
          tunnel: w281 -> [w314 _]
          tunnel: [w314 sgl[] [0.0, 0.0, 0.0] ("Traverse position (absolute, mm)")] -> w280
          tunnel: [w308 w339] -> w279
          tunnel: w278 -> [w309 _]
          tunnel: w270 -> [w311 _]
          tunnel: [w303 w338] -> w269
          tunnel: [w304 w332] -> w268
          tunnel: w267 -> [w305 _]
          tunnel: w266 -> [w303 w331]
          frame False {
            # "If traverse has not changed, but look-out radius has, then update it here."
            n60 = Subtract(x=w303, y=w311) -> (x-y=w307:sgl)
            n61 = Absolute Value(x=w307) -> (abs(x)=w313:sgl)
            n62 = Less?(x=w313, y=sgl 1.1920929e-07) -> (x < y?=w306:bool)
            n63 = case shown="False" w306 {
              tunnel: w309 -> [w322 w330]
              tunnel: [w321 w330] -> w308
              tunnel: w307 -> [w318 _]
              tunnel: w305 -> [w320 w329]
              tunnel: [w319 w329] -> w304
              frame False {
                n64 = in-place {
                  in-place-border: w318 -> [w326]
                  n65 = in-place-cluster #3(w322) -> ("Radius"=w328:sgl)
                  n66 = Add(x=w328, y=w326) -> (x+y=w327:sgl)
                  n67 = in-place-cluster #3("Radius"=w327) -> (w321:T8)
                }
                n68 = in-place {
                  in-place-border: w318 -> [w323]
                  n69 = in-place-cluster #4(w320) -> ("Radius"=w325:sgl)
                  n70 = Add(x=w325, y=w323) -> (x+y=w324:sgl)
                  n71 = in-place-cluster #4("Radius"=w324) -> (w319:T8)
                }
              }
              frame True {
              }
            }
          }
          frame True {
            n72 = global read "Collision Detection global.vi" "XYZ Components"() -> (w335:path)
            n73 = global read "Collision Detection global.vi" "XY Components"() -> (w336:path)
            n74 = global read "Collision Detection global.vi" "X Components"() -> (w337:path)
            n75 = call "Read triangles from stl file (binary format).vi"("STL file path"=w337) -> ("Triangles array"=w348:T7[], "Error out"=w346:errorcluster)  [unwired: 1 out]
            n76 = call "Read triangles from stl file (binary format).vi"("STL file path"=w336) -> ("Triangles array"=w333:T7[], "Error out"=w345:errorcluster)  [unwired: 1 out]
            n77 = call "Read triangles from stl file (binary format).vi"("STL file path"=w335) -> ("Triangles array"=w341:T7[], "Error out"=w344:errorcluster)  [unwired: 1 out]
            n78 = call "Creat bounding sphere.vi"("Triangles"=w341) -> ("Bounding sphere"=w340:T8)
            n79 = Merge Errors(w343, w346, w345, w344) -> (w347:errorcluster)
            n80 = call "Creat bounding sphere.vi"("Triangles"=w333) -> ("Bounding sphere"=w334:T8)
            n81 = in-place {
              in-place-border: [w352] -> w338
              in-place-border: w331 -> [w352]
              n82 = in-place-cluster #5(w340) -> ("Radius"=w354:sgl)
              n83 = Add(x=w354, y=w352) -> (x+y=w353:sgl)
              n84 = in-place-cluster #5("Radius"=w353) -> (w339:T8)
            }
            n85 = in-place {
              in-place-border: w331 -> [w349]
              n86 = in-place-cluster #6(w334) -> ("Radius"=w351:sgl)
              n87 = Add(x=w351, y=w349) -> (x+y=w350:sgl)
              n88 = in-place-cluster #6("Radius"=w350) -> (w332:T8)
            }
          }
        }
      }
      frame "Model rotation" {
        # "check if rotation axis coordinates have changed"
        # "check if rotation axis has changed (e.g from negation of angle)"
        # "check if rotation angle has changed"
        n89 = Subtract(x=w367, y=w364) -> (x-y=w366:sgl[])
        n90 = Subtract(x=w373, y=w374) -> (x-y=w397:sgl)
        n91 = Subtract(x=sgl 1.0, y=sgl 1.1920929e-07) -> (x-y=w368:sgl)
        n92 = call "Dot product.vi"("B"=w380, "A"=w375) -> ("A . B"=w379:sgl)
        n93 = call "Dot product.vi"("B"=w366, "A"=w366) -> ("A . B"=w370:sgl)
        n94 = Absolute Value(x=w397) -> (abs(x)=w405:sgl)
        n95 = Less?(x=w370, y=sgl 1.1920929e-07) -> (x < y?=w369:bool)
        n96 = Greater?(x=w379, y=w368) -> (0:w371:bool)
        n97 = Less?(x=w405, y=sgl 1.1920929e-07) -> (x < y?=w376:bool)
        n98 = And(x=w371, y=w369) -> (x .and. y?=w372:bool)
        n99 = Format Into String(format string="Traverse %s, Model %s", w359, w357) -> (resulting string=w358:string)  [unwired: 2 in, 1 out]
        n100 = case shown="False" w376 {
          tunnel: w398 -> [w422 w487]
          tunnel: w397 -> [w421 w486]
          tunnel: [w420 w485] -> w395
          tunnel: [w419 w484] -> w394
          tunnel: w393 -> [w418 w483]
          tunnel: [w417 w482] -> w390
          tunnel: w367 -> [w416 w481]
          tunnel: w380 -> [w415 w480]
          tunnel: w372 -> [w414 w479]
          tunnel: w374 -> [w413 w478]
          tunnel: w375 -> [w412 w477]
          tunnel: w373 -> [w411 w476]
          tunnel: w364 -> [w410 w475]
          tunnel: w358 -> [w409 w474]
          tunnel: w357 -> [w408 _]
          tunnel: w356 -> [w407 _]
          tunnel: w355 -> [w406 _]
          frame False {
            n101 = case shown="True" w414 {
              tunnel: w415 -> [w430 w461]
              tunnel: w422 -> [w428 _]
              tunnel: w421 -> [_ _]
              tunnel: w416 -> [w429 w462]
              tunnel: [w427 w458] -> w420
              tunnel: [w426 w459] -> w419
              tunnel: [w425 w457] -> w417
              tunnel: w418 -> [_ _]
              tunnel: w413 -> [w433 _]
              tunnel: w412 -> [w432 _]
              tunnel: w411 -> [w431 w460]
              tunnel: w410 -> [w424 _]
              tunnel: w409 -> [w423 w463]
              tunnel: w408 -> [_ w465]
              tunnel: w407 -> [_ w466]
              tunnel: w406 -> [_ w464]
              frame False {
                # "rotation axis has changed."
                # "re-build octree, and update arrays"
                # "rotate back to original state, then rotate by new angle about new axis"
                n102 = Negate(x=w433) -> (-x=w439:sgl)
                n103 = Multiply(x=w431, y=sgl 3.1415927) -> (x*y=w437:sgl)
                n104 = Multiply(x=w439, y=sgl 3.1415927) -> (x*y=w441:sgl)
                n105 = Divide(x=w437, y=sgl 180.0) -> (x/y=w438:sgl)
                n106 = Divide(x=w441, y=sgl 180.0) -> (x/y=w440:sgl)
                n107 = for {
                  tunnel: w428 -> [w456] mode=indexing
                  tunnel: w432 -> [w455]
                  tunnel: w440 -> [w454]
                  tunnel: [w452] -> w434 mode=indexing
                  tunnel: w424 -> [w453]
                  workers-P: _ -> [_]
                  n108 = call "Rotate triangle about arbitrary axis.vi"("Rotation angle (rad)"=w454, "Rotation axis coordinates (x, y, z)"=w453, "Rotation axis (unit direction vector)\nanti-clockwise positive looking into axis"=w455, "Triangle in"=w456) -> ("Triangle out"=w452:T7)
                }
                n109 = for {
                  tunnel: w434 -> [w451] mode=indexing
                  tunnel: w430 -> [w450]
                  tunnel: w438 -> [w449]
                  tunnel: [w447] -> w427 mode=indexing
                  tunnel: w429 -> [w448]
                  workers-P: _ -> [_]
                  n110 = call "Rotate triangle about arbitrary axis.vi"("Rotation angle (rad)"=w449, "Rotation axis coordinates (x, y, z)"=w448, "Rotation axis (unit direction vector)\nanti-clockwise positive looking into axis"=w450, "Triangle in"=w451) -> ("Triangle out"=w447:T7)
                }
                n111 = global read "Collision Detection global.vi" "Model octree resolution (model units)"() -> (w444:sgl)
                n112 = call "Get World extent.vi"("Triangles"=w427) -> ("Pmax (x, y, z)"=w445:sgl[], "Pmin (x, y, z)"=w446:sgl[])
                n113 = call "Build Octree from triangles.vi"("Octree resolution (model units)"=w444, "World Pmax (x, y, z)"=w445, "World Pmin (x, y, z)"=w446, "Triangle array"=w427, "String"=w423) -> ("Octree node array"=w426:T4[], "Stack error"=w425:errorcluster)  [unwired: 1 out]
              }
              frame True {
                n114 = global read "Collision Detection global.vi" "Model octree resolution (model units)"() -> (w469:sgl)
                n115 = Concatenate Strings(w465, ".stl" ("string")) -> (w467:string)
                n116 = Build Path(base path=w466, name or relative path="Model") -> (appended path=w472:path)
                n117 = Build Path(base path=w472, name or relative path=w467) -> (appended path=w470:path)
                n118 = call "Read stl file, build and save octree.vi"("STL file path (load)"=w470, "String"=w463, "Model rotation axis (unit vector)"=w461, "Auto resolution"=w464, "Specify resolution"=w469, "Invert model (interior region)"=FALSE, "Model Rotation (deg)"=w460, "Model rotation axis coordinates (absolute, mm)"=w462) -> ("Octree node array"=w459:T4[], "Error out"=w457:errorcluster, "Triangles array"=w458:T7[])  [unwired: 4 in, 1 out]
              }
            }
          }
          frame True {
            n119 = case shown="False" w479 {
              tunnel: w480 -> [w491 _]
              tunnel: w487 -> [w511 w522]
              tunnel: w486 -> [_ _]
              tunnel: w481 -> [w492 _]
              tunnel: [w490 w522] -> w485
              tunnel: [w508 w523] -> w484
              tunnel: [w507 errorcluster {"status"=FALSE, "code"=0, "source"=""} ("Stack error")] -> w482
              tunnel: w483 -> [_ w523]
              tunnel: w478 -> [w493 _]
              tunnel: w477 -> [w500 _]
              tunnel: w476 -> [w494 _]
              tunnel: w475 -> [w489 _]
              tunnel: w474 -> [w488 _]
              frame False {
                # "rotation axis has changed."
                # "re-build octree, and update arrays"
                # "rotate back to original state, then rotate by new angle about new axis"
                n120 = Negate(x=w493) -> (-x=w501:sgl)
                n121 = Multiply(x=w494, y=sgl 3.1415927) -> (x*y=w498:sgl)
                n122 = Multiply(x=w501, y=sgl 3.1415927) -> (x*y=w503:sgl)
                n123 = Divide(x=w498, y=sgl 180.0) -> (x/y=w499:sgl)
                n124 = Divide(x=w503, y=sgl 180.0) -> (x/y=w502:sgl)
                n125 = for {
                  tunnel: w511 -> [w521] mode=indexing
                  tunnel: w500 -> [w520]
                  tunnel: w502 -> [w519]
                  tunnel: [w517] -> w495 mode=indexing
                  tunnel: w489 -> [w518]
                  workers-P: _ -> [_]
                  n126 = call "Rotate triangle about arbitrary axis.vi"("Rotation angle (rad)"=w519, "Rotation axis coordinates (x, y, z)"=w518, "Rotation axis (unit direction vector)\nanti-clockwise positive looking into axis"=w520, "Triangle in"=w521) -> ("Triangle out"=w517:T7)
                }
                n127 = for {
                  tunnel: w495 -> [w516] mode=indexing
                  tunnel: w491 -> [w515]
                  tunnel: w499 -> [w514]
                  tunnel: [w512] -> w490 mode=indexing
                  tunnel: w492 -> [w513]
                  workers-P: _ -> [_]
                  n128 = call "Rotate triangle about arbitrary axis.vi"("Rotation angle (rad)"=w514, "Rotation axis coordinates (x, y, z)"=w513, "Rotation axis (unit direction vector)\nanti-clockwise positive looking into axis"=w515, "Triangle in"=w516) -> ("Triangle out"=w512:T7)
                }
                n129 = global read "Collision Detection global.vi" "Model octree resolution (model units)"() -> (w506:sgl)
                n130 = call "Get World extent.vi"("Triangles"=w490) -> ("Pmax (x, y, z)"=w509:sgl[], "Pmin (x, y, z)"=w510:sgl[])
                n131 = call "Build Octree from triangles.vi"("Octree resolution (model units)"=w506, "World Pmax (x, y, z)"=w509, "World Pmin (x, y, z)"=w510, "Triangle array"=w490, "String"=w488) -> ("Octree node array"=w508:T4[], "Stack error"=w507:errorcluster)  [unwired: 1 out]
              }
              frame True {
                # "no change, continue as is"
              }
            }
          }
        }
        n132 = Merge Errors(w391, w390) -> (w392:errorcluster)
      }
      frame "Traverse translation" {
        # "extrusion mode. Convex hull.\nPut original traverse into 'swap' shift register, and swap back after all collision detection checks"
        # "omit sqrt for speed"
        # "check if position has changed"
        n133 = Subtract(x=w545, y=w575) -> (x-y=w569:sgl[])
        n134 = call "Dot product.vi"("B"=w569, "A"=w569) -> ("A . B"=w553:sgl)
        n135 = Less?(x=w553, y=sgl 1.1920929e-07) -> (x < y?=w573:bool)
        n136 = case shown="False" w573 {
          tunnel: w572 -> [w645 w659]
          tunnel: w571 -> [w639 w658]
          tunnel: w570 -> [w638 w657]
          tunnel: w569 -> [w631 _]
          tunnel: [w637 w659] -> w544
          tunnel: [w636 w658] -> w543
          tunnel: [w635 w657] -> w542
          tunnel: w549 -> [w634 w656]
          tunnel: [w633 w656] -> w548
          tunnel: w526 -> [w632 w655]
          tunnel: [w630 w655] -> w525
          frame False {
            w641 = sgl 0.0 ("element")
            # "traverse has moved, translate triangles and update arrays as appropriate"
            n137 = Index Array(array=w631) -> (element=w644:sgl)  [unwired: 1 in]
            n138 = Index Array(array=w631) -> (element #1=w642:sgl, element #2=w643:sgl)  [unwired: 2 in]
            n139 = Build Array(w644, w641, w641) -> (w640:sgl[])
            n140 = Build Array(w642, w643, w641) -> (w629:sgl[])
            n141 = for {
              tunnel: w645 -> [w654] mode=indexing
              tunnel: w640 -> [w653]
              tunnel: [w652] -> w637 mode=indexing
              n142 = call "Translate triangle.vi"("Translation vector (dx, dy, dz)"=w653, "Triangle in"=w654) -> ("Triangle out"=w652:T7)
            }
            n143 = for {
              tunnel: w639 -> [w651] mode=indexing
              tunnel: w629 -> [w650]
              tunnel: [w649] -> w636 mode=indexing
              n144 = call "Translate triangle.vi"("Translation vector (dx, dy, dz)"=w650, "Triangle in"=w651) -> ("Triangle out"=w649:T7)
            }
            n145 = for {
              tunnel: w638 -> [w648] mode=indexing
              tunnel: w631 -> [w647]
              tunnel: [w646] -> w635 mode=indexing
              n146 = call "Translate triangle.vi"("Translation vector (dx, dy, dz)"=w647, "Triangle in"=w648) -> ("Triangle out"=w646:T7)
            }
            n147 = call "Translate sphere.vi"("Translation vector (dx, dy, dz)"=w631, "Sphere in"=w634) -> ("Sphere out"=w633:T8)
            n148 = call "Translate sphere.vi"("Translation vector (dx, dy, dz)"=w629, "Sphere in"=w632) -> ("Sphere out"=w630:T8)
          }
          frame True {
            # "no change, continue as is"
          }
        }
        n149 = case shown="True" w547 {
          tunnel: w542 -> [w578 w594]
          tunnel: [w578 w586] -> w539
          tunnel: w545 -> [_ w613]
          tunnel: w546 -> [_ w614]
          tunnel: w543 -> [w579 w597]
          tunnel: w544 -> [w580 w601]
          tunnel: [w579 w585] -> w540
          tunnel: [w580 w591] -> w541
          tunnel: [w577 w601] -> w536
          tunnel: [w577 w597] -> w537
          tunnel: [w577 w594] -> w538
          tunnel: [w576 TRUE] -> w529
          tunnel: w528 -> [w576 _]
          frame False {
            w577 = T7[] [] ("Triangles array")
          }
          frame True {
            w612 = sgl 0.0 ("element")
            n150 = Subtract(x=w614, y=w613) -> (x-y=w608:sgl[])
            n151 = Index Array(array=w608) -> (element=w609:sgl)  [unwired: 1 in]
            n152 = Index Array(array=w608) -> (element #1=w611:sgl, element #2=w610:sgl)  [unwired: 2 in]
            n153 = Build Array(w609, w612, w612) -> (w606:sgl[])
            n154 = Build Array(w611, w610, w612) -> (w607:sgl[])
            n155 = for {
              tunnel: w601 -> [w617] mode=indexing
              tunnel: w606 -> [w616]
              tunnel: [w615] -> w602 mode=indexing
              n156 = call "Translate triangle.vi"("Translation vector (dx, dy, dz)"=w616, "Triangle in"=w617) -> ("Triangle out"=w615:T7)
            }
            n157 = for {
              tunnel: w597 -> [w620] mode=indexing
              tunnel: w607 -> [w619]
              tunnel: [w618] -> w599 mode=indexing
              n158 = call "Translate triangle.vi"("Translation vector (dx, dy, dz)"=w619, "Triangle in"=w620) -> ("Triangle out"=w618:T7)
            }
            n159 = for {
              tunnel: w594 -> [w623] mode=indexing
              tunnel: w608 -> [w622]
              tunnel: [w621] -> w596 mode=indexing
              n160 = call "Translate triangle.vi"("Translation vector (dx, dy, dz)"=w622, "Triangle in"=w623) -> ("Triangle out"=w621:T7)
            }
            n161 = Build Array (concatenate)(w601, w602) -> (w600:T7[])
            n162 = Build Array (concatenate)(w597, w599) -> (w598:T7[])
            n163 = Build Array (concatenate)(w594, w596) -> (w595:T7[])
            n164 = call "Triangles to vertices (without duplicates).vi"("epsilon"=sgl 1.1920929e-07, "Triangles"=w600) -> ("Vertices (without duplicates)"=w603:sgl[][])
            n165 = call "Triangles to vertices (without duplicates).vi"("epsilon"=sgl 1.1920929e-07, "Triangles"=w598) -> ("Vertices (without duplicates)"=w604:sgl[][])
            n166 = call "Triangles to vertices (without duplicates).vi"("epsilon"=sgl 1.1920929e-07, "Triangles"=w595) -> ("Vertices (without duplicates)"=w605:sgl[][])
            n167 = call "Convex Hull 3D (GiftWrap).vi"("Vertices"=w603) -> ("Convex hull triangles, indexed"=w593:T9[])  [unwired: 1 out]
            n168 = call "Convex Hull 3D (GiftWrap).vi"("Vertices"=w604) -> ("Convex hull triangles, indexed"=w590:T9[])  [unwired: 1 out]
            n169 = call "Convex Hull 3D (GiftWrap).vi"("Vertices"=w605) -> ("Convex hull triangles, indexed"=w589:T9[])  [unwired: 1 out]
            n170 = call "Adapt triangles.vi"("Triangles in (indexed type)"=w593) -> ("Triangles out (full type)"=w592:T7[])
            n171 = call "Adapt triangles.vi"("Triangles in (indexed type)"=w590) -> ("Triangles out (full type)"=w588:T7[])
            n172 = call "Adapt triangles.vi"("Triangles in (indexed type)"=w589) -> ("Triangles out (full type)"=w587:T7[])
            n173 = call "Process adapted triangles (full).vi"("Triangles in"=w592) -> ("Triangles out"=w591:T7[])
            n174 = call "Process adapted triangles (full).vi"("Triangles in"=w588) -> ("Triangles out"=w585:T7[])
            n175 = call "Process adapted triangles (full).vi"("Triangles in"=w587) -> ("Triangles out"=w586:T7[])
          }
        }
        n176 = case shown="\"Traverse - Tunnel\"" w551 {
          tunnel: ["Tunnel Valid?" "Tunnel Valid?" "Model Valid?" "Fixed objects Valid?" "Traverse - Traverse Valid?"] -> w550
          frame "Traverse - Tunnel" {
          }
          frame "Traverse - All" {
          }
          frame "Traverse - Model" {
          }
          frame "Traverse - Fixed objects" {
          }
          frame "Traverse - Traverse" {
          }
        }
        n177 = Select(t="Render graphics", s=w560, f="End") -> (s? t:f=w558:string)
        n178 = Select(t=w558, s=w562, f=w550) -> (s? t:f=w561:string)
      }
      frame "Tunnel Valid?" {
        n179 = Array Size(array=w663) -> (size(s)=w662:i32)
        n180 = Greater Than 0?(x=w662) -> (x > 0?=w661:bool)
        n181 = Select(t="Collision detection: Traverse - Tunnel", s=w661, f="Model Valid?") -> (s? t:f=w694:string)
      }
      frame "Collision detection: Traverse - Tunnel" {
        # "Distinguish traverse part involved in collision"
        # "Only work with desired parts of traverse. Note XYZ is always checked(!)"
        # "If desired, and no collision, perform minimum separation test within sphere of influence"
        # "Checks traverse triangles against tunnel octree (and then triangles if necessary)"
        n182 = Unbundle By Name(w701) -> ("X"=w700:bool, "XY"=w699:bool, "XYZ"=w698:bool)
        n183 = case shown="False" w700 {
          tunnel: w744 -> [_ w778]
          tunnel: [sgl[][] [] ("Collision point(s)") w777] -> w733
          tunnel: [i32[] [] ("Indices of possible triangles") w776] -> w732
          tunnel: w722 -> [_ w775]
          tunnel: w721 -> [_ w774]
          tunnel: [FALSE w772] -> w709
          frame False {
          }
          frame True {
            n184 = for {
              tunnel: w778 -> [w788] mode=indexing
              tunnel: w774 -> [w787]
              tunnel: w775 -> [w786]
              tunnel: [w785] -> w777 mode=concatenating if=w780
              tunnel: [w783] -> w776 mode=concatenating if=w782
              shift-right: [w781] -> w772
              shift-left: FALSE -> [w779]
              n185 = call "Collision test simple.vi"("Octree for query triangles"=w786, "Query triangles"=w787, "Triangle to test"=w788) -> ("Indices of possible triangles"=w783:i32[], "Collision point(s)"=w785:sgl[][], "Collision(s)?"=w780:bool)
              n186 = Or(x=w779, y=w780) -> (x .or. y?=w781:bool)
              n187 = Empty Array?(array=w783) -> (empty?=w784:bool)
              n188 = Not(x=w784) -> (.not. x?=w782:bool)
            }
          }
        }
        n189 = case shown="False" w699 {
          tunnel: w743 -> [_ w798]
          tunnel: [sgl[][] [] ("Collision point(s)") w797] -> w735
          tunnel: [i32[] [] ("Indices of possible triangles") w796] -> w731
          tunnel: w722 -> [_ w795]
          tunnel: w721 -> [_ w794]
          tunnel: [FALSE w792] -> w708
          frame False {
          }
          frame True {
            n190 = for {
              tunnel: w798 -> [w808] mode=indexing
              tunnel: w794 -> [w807]
              tunnel: w795 -> [w806]
              tunnel: [w805] -> w797 mode=concatenating if=w800
              tunnel: [w803] -> w796 mode=concatenating if=w802
              shift-right: [w801] -> w792
              shift-left: FALSE ("Collision(s)?") -> [w799]
              n191 = call "Collision test simple.vi"("Octree for query triangles"=w806, "Query triangles"=w807, "Triangle to test"=w808) -> ("Indices of possible triangles"=w803:i32[], "Collision point(s)"=w805:sgl[][], "Collision(s)?"=w800:bool)
              n192 = Or(x=w799, y=w800) -> (x .or. y?=w801:bool)
              n193 = Empty Array?(array=w803) -> (empty?=w804:bool)
              n194 = Not(x=w804) -> (.not. x?=w802:bool)
            }
          }
        }
        n195 = case shown="True" w698 {
          tunnel: [sgl[][] [] ("Collision point(s)") w758] -> w734
          tunnel: [i32[] [] ("Indices of possible triangles") w757] -> w730
          tunnel: w723 -> [_ w756]
          tunnel: w722 -> [_ w755]
          tunnel: w721 -> [_ w754]
          tunnel: [FALSE w752] -> w703
          frame False {
          }
          frame True {
            n196 = for {
              tunnel: w756 -> [w768] mode=indexing
              tunnel: w754 -> [w767]
              tunnel: w755 -> [w766]
              tunnel: [w765] -> w758 mode=concatenating if=w761
              tunnel: [w763] -> w757 mode=concatenating if=w762
              shift-right: [w760] -> w752
              shift-left: FALSE ("Collision(s)?") -> [w759]
              n197 = call "Collision test simple.vi"("Octree for query triangles"=w766, "Query triangles"=w767, "Triangle to test"=w768) -> ("Indices of possible triangles"=w763:i32[], "Collision point(s)"=w765:sgl[][], "Collision(s)?"=w761:bool)
              n198 = Or(x=w759, y=w761) -> (x .or. y?=w760:bool)
              n199 = Empty Array?(array=w763) -> (empty?=w764:bool)
              n200 = Not(x=w764) -> (.not. x?=w762:bool)
            }
          }
        }
        n201 = Bundle(cluster=cluster{"X":bool, "XY":bool, "XYZ":bool} {"X"=FALSE, "XY"=FALSE, "XYZ"=FALSE} ("Traverse collision part"), "X"=w709, "XY"=w708, "XYZ"=w703) -> (w707:cluster{"X":bool, "XY":bool, "XYZ":bool})
        n202 = Compound Arithmetic op=OR(w709, w708, w703) -> (w716:bool)
        n203 = Build Array (concatenate)(w732, w731, w730) -> (w729:i32[])
        n204 = call "Remove duplicate indices.vi"("I32 array with duplicates"=w729) -> ("I32 array without duplicates"=w725:i32[])
        n205 = case shown="True" w716 {
          selector: w716 -> [w819 w821]
          tunnel: w735 -> [_ w825]
          tunnel: w734 -> [_ w824]
          tunnel: w733 -> [_ w823]
          tunnel: [sgl[][] [] w822] -> w737
          tunnel: [w819 w821] -> w728
          frame False {
          }
          frame True {
            n206 = Build Array (concatenate)(w823, w825, w824) -> (w822:sgl[][])
          }
        }
        n207 = Compound Arithmetic op=AND(invert w728, w727) -> (w726:bool)
        n208 = case shown="True" w726 {
          tunnel: [sgl 0.0 ("Minimum separation") w817] -> w740
          tunnel: [sgl[] [] ("Minimum separation vector\n(from all test triangles)") w818] -> w739
          tunnel: w725 -> [w811 _]
          tunnel: [w811 w816] -> w724
          tunnel: w723 -> [_ w815]
          tunnel: w720 -> [_ w814]
          tunnel: w722 -> [_ w813]
          tunnel: w721 -> [_ w812]
          frame False {
          }
          frame True {
            n209 = call "Get minimum separation within sphere.vi"("Triangles to test"=w815, "Query triangles"=w812, "Octree for query triangles"=w813, "Sphere of interest"=w814) -> ("Minimum separation vector\n(from all test triangles)"=w818:sgl[], "Minimum separation"=w817:sgl, "Indices of possible triangles"=w816:i32[])  [unwired: 2 in]
          }
        }
      }
      frame "Model Valid?" {
        n210 = Array Size(array=w827) -> (size(s)=w829:i32)
        n211 = Greater Than 0?(x=w829) -> (x > 0?=w828:bool)
        n212 = Select(t="Collision detection: Traverse - Model", s=w828, f="Fixed objects Valid?") -> (s? t:f=w860:string)
      }
      frame "Collision detection: Traverse - Model" {
        # "Distinguish traverse part involved in collision"
        # "Only work with desired parts of traverse."
        # "append to existing values in case of \"all\" collision mode"
        # "Checks traverse triangles against model octree (and then triangles if necessary)"
        n213 = Unbundle By Name(w881) -> ("X"=w880:bool, "XY"=w871:bool, "XYZ"=w869:bool)
        n214 = case shown="True" w880 {
          tunnel: w927 -> [w1037 _]
          tunnel: [w1036 sgl[][] [] ("Collision point(s)")] -> w914
          tunnel: [w1035 i32[] [] ("Indices of possible triangles")] -> w911
          tunnel: w865 -> [w1034 _]
          tunnel: w878 -> [w1033 _]
          tunnel: [w1032 FALSE] -> w887
          frame True {
            n215 = for {
              tunnel: w1037 -> [w1047] mode=indexing
              tunnel: w1034 -> [w1046]
              tunnel: w1033 -> [w1045]
              tunnel: [w1044] -> w1036 mode=concatenating if=w1039
              tunnel: [w1042] -> w1035 mode=concatenating if=w1041
              shift-right: [w1040] -> w1032
              shift-left: FALSE -> [w1038]
              n216 = call "Collision test simple.vi"("Octree for query triangles"=w1045, "Query triangles"=w1046, "Triangle to test"=w1047) -> ("Indices of possible triangles"=w1042:i32[], "Collision point(s)"=w1044:sgl[][], "Collision(s)?"=w1039:bool)
              n217 = Or(x=w1038, y=w1039) -> (x .or. y?=w1040:bool)
              n218 = Empty Array?(array=w1042) -> (empty?=w1043:bool)
              n219 = Not(x=w1043) -> (.not. x?=w1041:bool)
            }
          }
          frame False {
          }
        }
        n220 = case shown="True" w871 {
          tunnel: w873 -> [_ w1020]
          tunnel: [sgl[][] [] ("Collision point(s)") w1019] -> w913
          tunnel: [i32[] [] ("Indices of possible triangles") w1018] -> w910
          tunnel: w865 -> [_ w1017]
          tunnel: w878 -> [_ w1016]
          tunnel: [FALSE w1015] -> w886
          frame False {
          }
          frame True {
            n221 = for {
              tunnel: w1020 -> [w1030] mode=indexing
              tunnel: w1017 -> [w1029]
              tunnel: w1016 -> [w1028]
              tunnel: [w1027] -> w1019 mode=concatenating if=w1022
              tunnel: [w1025] -> w1018 mode=concatenating if=w1024
              shift-right: [w1023] -> w1015
              shift-left: FALSE -> [w1021]
              n222 = call "Collision test simple.vi"("Octree for query triangles"=w1028, "Query triangles"=w1029, "Triangle to test"=w1030) -> ("Indices of possible triangles"=w1025:i32[], "Collision point(s)"=w1027:sgl[][], "Collision(s)?"=w1022:bool)
              n223 = Or(x=w1021, y=w1022) -> (x .or. y?=w1023:bool)
              n224 = Empty Array?(array=w1025) -> (empty?=w1026:bool)
              n225 = Not(x=w1026) -> (.not. x?=w1024:bool)
            }
          }
        }
        n226 = case shown="True" w869 {
          tunnel: [sgl[][] [] ("Collision point(s)") w1000] -> w912
          tunnel: [i32[] [] ("Indices of possible triangles") w999] -> w909
          tunnel: w877 -> [_ w998]
          tunnel: w878 -> [_ w997]
          tunnel: w865 -> [_ w996]
          tunnel: [FALSE w994] -> w882
          frame False {
          }
          frame True {
            n227 = for {
              tunnel: w998 -> [w1010] mode=indexing
              tunnel: w996 -> [w1009]
              tunnel: w997 -> [w1008]
              tunnel: [w1007] -> w1000 mode=concatenating if=w1001
              tunnel: [w1005] -> w999 mode=concatenating if=w1004
              shift-right: [w1003] -> w994
              shift-left: FALSE -> [w1002]
              n228 = call "Collision test simple.vi"("Octree for query triangles"=w1008, "Query triangles"=w1009, "Triangle to test"=w1010) -> ("Indices of possible triangles"=w1005:i32[], "Collision point(s)"=w1007:sgl[][], "Collision(s)?"=w1001:bool)
              n229 = Or(x=w1002, y=w1001) -> (x .or. y?=w1003:bool)
              n230 = Empty Array?(array=w1005) -> (empty?=w1006:bool)
              n231 = Not(x=w1006) -> (.not. x?=w1004:bool)
            }
          }
        }
        n232 = Unbundle(w894) -> ("X"=w891:bool, "XY"=w892:bool, "XYZ"=w893:bool)
        n233 = Or(x=w882, y=w893) -> (x .or. y?=w888:bool)
        n234 = Or(x=w886, y=w892) -> (x .or. y?=w889:bool)
        n235 = Compound Arithmetic op=OR(w887, w886, w882) -> (w901:bool)
        n236 = Build Array (concatenate)(w911, w910, w909) -> (w908:i32[])
        n237 = Or(x=w887, y=w891) -> (x .or. y?=w890:bool)
        n238 = Bundle(cluster=w894, "X"=w890, "XY"=w889, "XYZ"=w888) -> (w885:cluster{"X":bool, "XY":bool, "XYZ":bool})
        n239 = Empty Array?(array=w865) -> (empty?=w864:bool)
        n240 = case shown="False" w901 {
          selector: w901 -> [w1052 w1053]
          tunnel: w914 -> [_ w1057]
          tunnel: w913 -> [_ w1056]
          tunnel: w912 -> [_ w1055]
          tunnel: [sgl[][] [] w1054] -> w915
          tunnel: [w1052 w1053] -> w917
          frame False {
          }
          frame True {
            n241 = Build Array (concatenate)(w1057, w1056, w1055) -> (w1054:sgl[][])
          }
        }
        n242 = call "Remove duplicate indices.vi"("I32 array with duplicates"=w908) -> ("I32 array without duplicates"=w876:i32[])
        n243 = Or(x=w917, y=w916) -> (x .or. y?=w907:bool)
        n244 = Compound Arithmetic op=AND(invert w864, invert w907, w906) -> (w870:bool)
        n245 = case shown="False" w870 {
          tunnel: [w933 w950] -> w866
          tunnel: [w934 w952] -> w868
          tunnel: w876 -> [w937 w941]
          tunnel: [w937 w947] -> w867
          tunnel: w877 -> [_ w964]
          tunnel: w879 -> [_ w963]
          tunnel: w878 -> [_ w960]
          tunnel: w865 -> [_ w961]
          tunnel: w875 -> [w935 w942]
          tunnel: w874 -> [w936 w943]
          tunnel: w873 -> [_ w962]
          tunnel: w872 -> [_ w959]
          tunnel: w871 -> [_ w955]
          tunnel: w869 -> [_ w954]
          tunnel: w864 -> [w932 _]
          frame False {
            n246 = case shown="True" w932 {
              tunnel: w936 -> [_ w940]
              tunnel: [_ w940] -> w934
              tunnel: [sgl 0.0 ("Minimum separation") w939] -> w933
              tunnel: w935 -> [_ w939]
              frame False {
              }
              frame True {
              }
            }
          }
          frame True {
            n247 = case shown="False" w954 {
              tunnel: w964 -> [_ w980]
              tunnel: w963 -> [_ w979]
              tunnel: w961 -> [_ w978]
              tunnel: w960 -> [_ w977]
              tunnel: [w972 w976] -> w946
              tunnel: [w973 w975] -> w945
              tunnel: [w971 w974] -> w944
              tunnel: w943 -> [w973 _]
              tunnel: w942 -> [w972 _]
              tunnel: w941 -> [w971 _]
              frame False {
              }
              frame True {
                n248 = call "Get minimum separation within sphere.vi"("Triangles to test"=w980, "Query triangles"=w978, "Octree for query triangles"=w977, "Sphere of interest"=w979) -> ("Minimum separation vector\n(from all test triangles)"=w975:sgl[], "Minimum separation"=w976:sgl, "Indices of possible triangles"=w974:i32[])  [unwired: 2 in]
              }
            }
            n249 = case shown="False" w955 {
              tunnel: w962 -> [_ w990]
              tunnel: w961 -> [_ w989]
              tunnel: w960 -> [_ w988]
              tunnel: w959 -> [_ w987]
              tunnel: [w982 w986] -> w949
              tunnel: [w983 w985] -> w951
              tunnel: [w981 w984] -> w948
              tunnel: w943 -> [w983 _]
              tunnel: w942 -> [w982 _]
              tunnel: w941 -> [w981 _]
              frame False {
              }
              frame True {
                n250 = call "Get minimum separation within sphere.vi"("Triangles to test"=w990, "Query triangles"=w989, "Octree for query triangles"=w988, "Sphere of interest"=w987) -> ("Minimum separation vector\n(from all test triangles)"=w985:sgl[], "Minimum separation"=w986:sgl, "Indices of possible triangles"=w984:i32[])  [unwired: 2 in]
              }
            }
            n251 = Less?(x=w949, y=w946) -> (x < y?=w957:bool)
            n252 = Greater?(x=w949, y=sgl 0.001) -> (0:w956:bool)
            n253 = And(x=w956, y=w957) -> (x .and. y?=w953:bool)
            n254 = case shown="False" w953 {
              tunnel: [w966 w970] -> w952
              tunnel: w951 -> [_ w970]
              tunnel: [w967 w969] -> w950
              tunnel: w949 -> [_ w969]
              tunnel: w948 -> [_ w968]
              tunnel: [w965 w968] -> w947
              tunnel: w946 -> [w967 _]
              tunnel: w945 -> [w966 _]
              tunnel: w944 -> [w965 _]
              frame False {
              }
              frame True {
              }
            }
          }
        }
        n255 = Less?(x=w866, y=w875) -> (x < y?=w921:bool)
        n256 = case shown="True" w921 {
          tunnel: w875 -> [w1058 _]
          tunnel: w866 -> [_ w1060]
          tunnel: [w1058 w1060] -> w920
          tunnel: w868 -> [_ w1061]
          tunnel: [w1059 w1061] -> w919
          tunnel: w874 -> [w1059 _]
          frame False {
          }
          frame True {
          }
        }
        n257 = Build Array (concatenate)(w902, w915) -> (w922:sgl[][])
      }
      frame "Fixed objects Valid?" {
        n258 = Array Size(array=w1063) -> (size(s)=w1066:i32)
        n259 = Greater Than 0?(x=w1066) -> (x > 0?=w1065:bool)
        n260 = Select(t="Collision detection: Traverse - Fixed objects", s=w1065, f="Collision detection: Traverse - Traverse") -> (s? t:f=w1096:string)
      }
      frame "Collision detection: Traverse - Fixed objects" {
        # "Distinguish traverse part involved in collision"
        # "Only work with desired parts of traverse."
        # "append to existing values in case of \"all\" collision mode"
        # "Checks traverse triangles against fixed objects octree (and then triangles if necessary)"
        n261 = Unbundle By Name(w1117) -> ("X"=w1116:bool, "XY"=w1101:bool, "XYZ"=w1100:bool)
        n262 = case shown="False" w1116 {
          tunnel: w1164 -> [w1274 _]
          tunnel: [w1273 sgl[][] [] ("Collision point(s)")] -> w1151
          tunnel: [w1272 i32[] [] ("Indices of possible triangles")] -> w1148
          tunnel: w1114 -> [w1271 _]
          tunnel: w1113 -> [w1270 _]
          tunnel: [w1269 FALSE] -> w1122
          frame True {
            n263 = for {
              tunnel: w1274 -> [w1284] mode=indexing
              tunnel: w1271 -> [w1283]
              tunnel: w1270 -> [w1282]
              tunnel: [w1281] -> w1273 mode=concatenating if=w1277
              tunnel: [w1279] -> w1272 mode=concatenating if=w1278
              shift-right: [w1275] -> w1269
              shift-left: FALSE -> [w1276]
              n264 = call "Collision test simple.vi"("Octree for query triangles"=w1282, "Query triangles"=w1283, "Triangle to test"=w1284) -> ("Indices of possible triangles"=w1279:i32[], "Collision point(s)"=w1281:sgl[][], "Collision(s)?"=w1277:bool)
              n265 = Or(x=w1276, y=w1277) -> (x .or. y?=w1275:bool)
              n266 = Empty Array?(array=w1279) -> (empty?=w1280:bool)
              n267 = Not(x=w1280) -> (.not. x?=w1278:bool)
            }
          }
          frame False {
          }
        }
        n268 = case shown="False" w1101 {
          tunnel: w1111 -> [_ w1257]
          tunnel: [sgl[][] [] ("Collision point(s)") w1256] -> w1150
          tunnel: [i32[] [] ("Indices of possible triangles") w1255] -> w1147
          tunnel: w1114 -> [_ w1254]
          tunnel: w1113 -> [_ w1253]
          tunnel: [FALSE w1252] -> w1121
          frame False {
          }
          frame True {
            n269 = for {
              tunnel: w1257 -> [w1267] mode=indexing
              tunnel: w1254 -> [w1266]
              tunnel: w1253 -> [w1265]
              tunnel: [w1264] -> w1256 mode=concatenating if=w1259
              tunnel: [w1262] -> w1255 mode=concatenating if=w1261
              shift-right: [w1260] -> w1252
              shift-left: FALSE -> [w1258]
              n270 = call "Collision test simple.vi"("Octree for query triangles"=w1265, "Query triangles"=w1266, "Triangle to test"=w1267) -> ("Indices of possible triangles"=w1262:i32[], "Collision point(s)"=w1264:sgl[][], "Collision(s)?"=w1259:bool)
              n271 = Or(x=w1258, y=w1259) -> (x .or. y?=w1260:bool)
              n272 = Empty Array?(array=w1262) -> (empty?=w1263:bool)
              n273 = Not(x=w1263) -> (.not. x?=w1261:bool)
            }
          }
        }
        n274 = case shown="True" w1100 {
          tunnel: [sgl[][] [] ("Collision point(s)") w1237] -> w1149
          tunnel: [i32[] [] ("Indices of possible triangles") w1236] -> w1146
          tunnel: w1115 -> [_ w1235]
          tunnel: w1113 -> [_ w1234]
          tunnel: w1114 -> [_ w1233]
          tunnel: [FALSE w1231] -> w1118
          frame False {
          }
          frame True {
            n275 = for {
              tunnel: w1235 -> [w1247] mode=indexing
              tunnel: w1233 -> [w1246]
              tunnel: w1234 -> [w1245]
              tunnel: [w1244] -> w1237 mode=concatenating if=w1240
              tunnel: [w1242] -> w1236 mode=concatenating if=w1241
              shift-right: [w1238] -> w1231
              shift-left: FALSE -> [w1239]
              n276 = call "Collision test simple.vi"("Octree for query triangles"=w1245, "Query triangles"=w1246, "Triangle to test"=w1247) -> ("Indices of possible triangles"=w1242:i32[], "Collision point(s)"=w1244:sgl[][], "Collision(s)?"=w1240:bool)
              n277 = Or(x=w1239, y=w1240) -> (x .or. y?=w1238:bool)
              n278 = Empty Array?(array=w1242) -> (empty?=w1243:bool)
              n279 = Not(x=w1243) -> (.not. x?=w1241:bool)
            }
          }
        }
        n280 = Unbundle(w1124) -> ("X"=w1128:bool, "XY"=w1129:bool, "XYZ"=w1130:bool)
        n281 = Or(x=w1118, y=w1130) -> (x .or. y?=w1125:bool)
        n282 = Or(x=w1121, y=w1129) -> (x .or. y?=w1126:bool)
        n283 = Compound Arithmetic op=OR(w1122, w1121, w1118) -> (w1136:bool)
        n284 = Build Array (concatenate)(w1148, w1147, w1146) -> (w1145:i32[])
        n285 = Or(x=w1122, y=w1128) -> (x .or. y?=w1127:bool)
        n286 = Bundle(cluster=w1124, "X"=w1127, "XY"=w1126, "XYZ"=w1125) -> (w1123:cluster{"X":bool, "XY":bool, "XYZ":bool})
        n287 = case shown="True" w1136 {
          selector: w1136 -> [w1289 w1290]
          tunnel: w1151 -> [_ w1294]
          tunnel: w1150 -> [_ w1293]
          tunnel: w1149 -> [_ w1292]
          tunnel: [sgl[][] [] w1291] -> w1152
          tunnel: [w1289 w1290] -> w1154
          frame False {
          }
          frame True {
            n288 = Build Array (concatenate)(w1294, w1293, w1292) -> (w1291:sgl[][])
          }
        }
        n289 = call "Remove duplicate indices.vi"("I32 array with duplicates"=w1145) -> ("I32 array without duplicates"=w1105:i32[])
        n290 = Empty Array?(array=w1114) -> (empty?=w1109:bool)
        n291 = Or(x=w1154, y=w1153) -> (x .or. y?=w1144:bool)
        n292 = Compound Arithmetic op=AND(invert w1109, invert w1144, w1141) -> (w1102:bool)
        n293 = case shown="False" w1102 {
          tunnel: [w1169 w1187] -> w1107
          tunnel: [w1170 w1189] -> w1108
          tunnel: w1105 -> [w1174 w1178]
          tunnel: [w1174 w1184] -> w1106
          tunnel: w1115 -> [_ w1201]
          tunnel: w1112 -> [_ w1200]
          tunnel: w1113 -> [_ w1197]
          tunnel: w1114 -> [_ w1198]
          tunnel: w1103 -> [w1171 w1179]
          tunnel: w1104 -> [w1172 w1180]
          tunnel: w1109 -> [w1173 _]
          tunnel: w1111 -> [_ w1199]
          tunnel: w1110 -> [_ w1196]
          tunnel: w1101 -> [_ w1192]
          tunnel: w1100 -> [_ w1191]
          frame False {
            n294 = case shown="True" w1173 {
              tunnel: w1172 -> [_ w1177]
              tunnel: [_ w1177] -> w1170
              tunnel: [sgl 0.0 ("Minimum separation") w1176] -> w1169
              tunnel: w1171 -> [_ w1176]
              frame False {
              }
              frame True {
              }
            }
          }
          frame True {
            n295 = case shown="False" w1191 {
              tunnel: w1201 -> [_ w1217]
              tunnel: w1200 -> [_ w1216]
              tunnel: w1198 -> [_ w1215]
              tunnel: w1197 -> [_ w1214]
              tunnel: [w1209 w1213] -> w1183
              tunnel: [w1210 w1212] -> w1182
              tunnel: [w1208 w1211] -> w1181
              tunnel: w1180 -> [w1210 _]
              tunnel: w1179 -> [w1209 _]
              tunnel: w1178 -> [w1208 _]
              frame False {
              }
              frame True {
                n296 = call "Get minimum separation within sphere.vi"("Triangles to test"=w1217, "Query triangles"=w1215, "Octree for query triangles"=w1214, "Sphere of interest"=w1216) -> ("Minimum separation vector\n(from all test triangles)"=w1212:sgl[], "Minimum separation"=w1213:sgl, "Indices of possible triangles"=w1211:i32[])  [unwired: 2 in]
              }
            }
            n297 = case shown="False" w1192 {
              tunnel: w1199 -> [_ w1227]
              tunnel: w1198 -> [_ w1226]
              tunnel: w1197 -> [_ w1225]
              tunnel: w1196 -> [_ w1224]
              tunnel: [w1219 w1223] -> w1186
              tunnel: [w1220 w1222] -> w1188
              tunnel: [w1218 w1221] -> w1185
              tunnel: w1180 -> [w1220 _]
              tunnel: w1179 -> [w1219 _]
              tunnel: w1178 -> [w1218 _]
              frame False {
              }
              frame True {
                n298 = call "Get minimum separation within sphere.vi"("Triangles to test"=w1227, "Query triangles"=w1226, "Octree for query triangles"=w1225, "Sphere of interest"=w1224) -> ("Minimum separation vector\n(from all test triangles)"=w1222:sgl[], "Minimum separation"=w1223:sgl, "Indices of possible triangles"=w1221:i32[])  [unwired: 2 in]
              }
            }
            n299 = Less?(x=w1186, y=w1183) -> (x < y?=w1194:bool)
            n300 = Greater?(x=w1186, y=sgl 0.001) -> (0:w1193:bool)
            n301 = And(x=w1193, y=w1194) -> (x .and. y?=w1190:bool)
            n302 = case shown="False" w1190 {
              tunnel: [w1203 w1207] -> w1189
              tunnel: w1188 -> [_ w1207]
              tunnel: [w1204 w1206] -> w1187
              tunnel: w1186 -> [_ w1206]
              tunnel: w1185 -> [_ w1205]
              tunnel: [w1202 w1205] -> w1184
              tunnel: w1183 -> [w1204 _]
              tunnel: w1182 -> [w1203 _]
              tunnel: w1181 -> [w1202 _]
              frame False {
              }
              frame True {
              }
            }
          }
        }
        n303 = Less?(x=w1107, y=w1103) -> (x < y?=w1158:bool)
        n304 = Build Array (concatenate)(w1137, w1152) -> (w1159:sgl[][])
        n305 = case shown="True" w1158 {
          tunnel: w1103 -> [w1295 _]
          tunnel: w1107 -> [_ w1297]
          tunnel: [w1295 w1297] -> w1157
          tunnel: w1108 -> [_ w1298]
          tunnel: [w1296 w1298] -> w1156
          tunnel: w1104 -> [w1296 _]
          frame False {
          }
          frame True {
          }
        }
      }
      frame "Collision detection: Traverse - Traverse" {
        # "NOT YET IMPLEMENTED!"
        n306 = Select(t="Render graphics", s=w1331, f="End") -> (s? t:f=w1330:string)
      }
      frame "Render graphics" {
        w1364 = T3 {"Red"=0.66, "Green"=0.5, "Blue"=0.5, "Alpha"=1.0} ("Colour")
        w1354 = T3 {"Red"=0.25, "Green"=0.25, "Blue"=0.25, "Alpha"=1.0} ("Colour")
        w1351 = T10."Polygons" ("Render mode")
        # "Critical to close this reference to prevent serious memory leak!"
        n307 = Empty Array?(array=w1385) -> (empty?=w1384:bool)
        n308 = Not(x=w1384) -> (.not. x?=w1383:bool)
        n309 = global read "Collision Detection global.vi" "Draw octree leaf-node boxes"() -> (w1371:bool)
        n310 = global read "Collision Detection global.vi" "Highlight tested triangles"() -> (w1347:bool)
        n311 = And(x=w1383, y=w1347) -> (x .and. y?=w1382:bool)
        n312 = case shown="True" w1382 {
          tunnel: w1410 -> [w1484 w1488]
          tunnel: T3 {"Red"=1.0, "Green"=1.0, "Blue"=1.0, "Alpha"=1.0} ("Colour") -> [w1483 w1497]
          tunnel: w1351 -> [w1482 w1496]
          tunnel: [w1481 w1490] -> w1401
          tunnel: [w1479 w1495] -> w1386
          tunnel: w1385 -> [_ w1485]
          frame False {
            n313 = call "Create triangles mesh.vi"("Colour"=w1483, "Render mode"=w1482, "Triangles array"=w1484) -> ("Error out"=w1481:errorcluster, "Triangle mesh out"=w1480:refnum<vi>)
            n314 = Build Array(w1480) -> (w1479:refnum<vi>[])
          }
          frame True {
            n315 = for {
              tunnel: [w1501] -> w1486 mode=indexing if=w1499
              tunnel: w1488 -> [w1501] mode=indexing
              tunnel: w1485 -> [w1504]
              shift-right: [w1502] -> _
              shift-left: 0 -> [w1503]
              tunnel: [w1501] -> w1487 mode=indexing if=w1500
              i -> [w1506]
              n316 = Index Array(array=w1504, index=w1503) -> (element=w1505:i32)
              n317 = Equal?(x=w1505, y=w1506) -> (x = y?=w1499:bool)
              n318 = case shown="True" w1499 {
                tunnel: w1503 -> [w1507 w1509]
                tunnel: [w1507 w1508] -> w1502
                frame False {
                }
                frame True {
                  n319 = Increment(x=w1509) -> (x+1=w1508:i32)
                }
              }
              n320 = Not(x=w1499) -> (.not. x?=w1500:bool)
            }
            n321 = call "Create triangles mesh.vi"("Colour"=w1497, "Render mode"=w1496, "Triangles array"=w1487) -> ("Error out"=w1492:errorcluster, "Triangle mesh out"=w1494:refnum<vi>)
            n322 = call "Create triangles mesh.vi"("Colour"=T3 {"Red"=0.75, "Green"=1.0, "Blue"=1.0, "Alpha"=1.0}, "Render mode"=w1496, "Triangles array"=w1486) -> ("Error out"=w1491:errorcluster, "Triangle mesh out"=w1493:refnum<vi>)
            n323 = Build Array(w1494, w1493) -> (w1495:refnum<vi>[])
            n324 = Merge Errors(w1492, w1491) -> (w1490:errorcluster)
          }
        }
        n325 = Empty Array?(array=w1345) -> (empty?=w1380:bool)
        n326 = Not(x=w1380) -> (.not. x?=w1381:bool)
        n327 = And(x=w1381, y=w1347) -> (x .and. y?=w1366:bool)
        n328 = case shown="True" w1366 {
          tunnel: w1368 -> [w1453 w1457]
          tunnel: w1354 -> [w1452 w1466]
          tunnel: w1351 -> [w1451 w1465]
          tunnel: [w1450 w1459] -> w1365
          tunnel: [w1448 w1464] -> w1367
          tunnel: w1345 -> [_ w1454]
          frame False {
            n329 = call "Create triangles mesh.vi"("Colour"=w1452, "Render mode"=w1451, "Triangles array"=w1453) -> ("Error out"=w1450:errorcluster, "Triangle mesh out"=w1449:refnum<vi>)
            n330 = Build Array(w1449) -> (w1448:refnum<vi>[])
          }
          frame True {
            n331 = for {
              tunnel: [w1470] -> w1456 mode=indexing if=w1468
              tunnel: w1457 -> [w1470] mode=indexing
              tunnel: w1454 -> [w1473]
              shift-right: [w1471] -> _
              shift-left: 0 -> [w1472]
              tunnel: [w1470] -> w1455 mode=indexing if=w1469
              i -> [w1475]
              n332 = Index Array(array=w1473, index=w1472) -> (element=w1474:i32)
              n333 = Equal?(x=w1474, y=w1475) -> (x = y?=w1468:bool)
              n334 = case shown="True" w1468 {
                tunnel: w1472 -> [w1476 w1478]
                tunnel: [w1476 w1477] -> w1471
                frame False {
                }
                frame True {
                  n335 = Increment(x=w1478) -> (x+1=w1477:i32)
                }
              }
              n336 = Not(x=w1468) -> (.not. x?=w1469:bool)
            }
            n337 = call "Create triangles mesh.vi"("Colour"=w1466, "Render mode"=w1465, "Triangles array"=w1455) -> ("Error out"=w1461:errorcluster, "Triangle mesh out"=w1463:refnum<vi>)
            n338 = call "Create triangles mesh.vi"("Colour"=T3 {"Red"=1.0, "Green"=0.85, "Blue"=0.0, "Alpha"=1.0}, "Render mode"=w1465, "Triangles array"=w1456) -> ("Error out"=w1460:errorcluster, "Triangle mesh out"=w1462:refnum<vi>)
            n339 = Build Array(w1463, w1462) -> (w1464:refnum<vi>[])
            n340 = Merge Errors(w1461, w1460) -> (w1459:errorcluster)
          }
        }
        n341 = Empty Array?(array=w1344) -> (empty?=w1349:bool)
        n342 = Not(x=w1349) -> (.not. x?=w1348:bool)
        n343 = And(x=w1348, y=w1347) -> (x .and. y?=w1346:bool)
        n344 = case shown="True" w1346 {
          tunnel: w1352 -> [w1422 w1425]
          tunnel: w1354 -> [w1421 w1435]
          tunnel: w1351 -> [w1420 w1434]
          tunnel: [w1419 w1428] -> w1350
          tunnel: [w1417 w1433] -> w1353
          tunnel: w1344 -> [_ w1426]
          frame False {
            n345 = call "Create triangles mesh.vi"("Colour"=w1421, "Render mode"=w1420, "Triangles array"=w1422) -> ("Error out"=w1419:errorcluster, "Triangle mesh out"=w1418:refnum<vi>)
            n346 = Build Array(w1418) -> (w1417:refnum<vi>[])
          }
          frame True {
            n347 = for {
              tunnel: [w1439] -> w1424 mode=indexing if=w1437
              tunnel: w1425 -> [w1439] mode=indexing
              tunnel: w1426 -> [w1442]
              shift-right: [w1440] -> _
              shift-left: 0 -> [w1441]
              tunnel: [w1439] -> w1423 mode=indexing if=w1438
              i -> [w1444]
              n348 = Index Array(array=w1442, index=w1441) -> (element=w1443:i32)
              n349 = Equal?(x=w1443, y=w1444) -> (x = y?=w1437:bool)
              n350 = case shown="True" w1437 {
                tunnel: w1441 -> [w1445 w1447]
                tunnel: [w1445 w1446] -> w1440
                frame False {
                }
                frame True {
                  n351 = Increment(x=w1447) -> (x+1=w1446:i32)
                }
              }
              n352 = Not(x=w1437) -> (.not. x?=w1438:bool)
            }
            n353 = call "Create triangles mesh.vi"("Colour"=w1435, "Render mode"=w1434, "Triangles array"=w1423) -> ("Error out"=w1430:errorcluster, "Triangle mesh out"=w1432:refnum<vi>)
            n354 = call "Create triangles mesh.vi"("Colour"=T3 {"Red"=1.0, "Green"=0.85, "Blue"=0.0, "Alpha"=1.0}, "Render mode"=w1434, "Triangles array"=w1424) -> ("Error out"=w1429:errorcluster, "Triangle mesh out"=w1431:refnum<vi>)
            n355 = Build Array(w1432, w1431) -> (w1433:refnum<vi>[])
            n356 = Merge Errors(w1430, w1429) -> (w1428:errorcluster)
          }
        }
        n357 = call "Create triangles mesh.vi"("Colour"=w1364, "Render mode"=w1351, "Triangles array"=w1409) -> ("Error out"=w1400:errorcluster, "Triangle mesh out"=w1392:refnum<vi>)
        n358 = call "Create triangles mesh.vi"("Colour"=w1364, "Render mode"=w1351, "Triangles array"=w1408) -> ("Error out"=w1399:errorcluster, "Triangle mesh out"=w1391:refnum<vi>)
        n359 = call "Create triangles mesh.vi"("Colour"=w1364, "Render mode"=w1351, "Triangles array"=w1407) -> ("Error out"=w1398:errorcluster, "Triangle mesh out"=w1390:refnum<vi>)
        n360 = Build Array (concatenate)(w1386, w1367, w1353, w1392, w1391, w1390) -> (w1378:refnum<vi>[])
        n361 = case shown="True" w1371 {
          tunnel: w1406 -> [_ w1534]
          tunnel: w1405 -> [_ w1533]
          tunnel: T3 {"Red"=0.0, "Green"=0.25, "Blue"=0.0, "Alpha"=1.0} ("Colour (emission)") -> [_ w1530]
          tunnel: T3 {"Red"=0.0, "Green"=0.5, "Blue"=0.5, "Alpha"=1.0} ("Colour (emission)") -> [_ w1529]
          tunnel: [errorcluster {"status"=FALSE, "code"=0, "source"=""} ("error IO") w1523] -> w1397
          tunnel: [w1521 w1522] -> w1377
          tunnel: w1378 -> [w1521 w1526]
          frame False {
          }
          frame True {
            n362 = call "Create Octree node boxes.vi"("Colour (emission)"=w1530, "Draw populated leaf nodes only"=TRUE, "Octree nodes array"=w1534) -> ("Error out"=w1525:errorcluster, "Octree node boxes array"=w1528:refnum<vi>[])
            n363 = call "Create Octree node boxes.vi"("Colour (emission)"=w1529, "Draw populated leaf nodes only"=TRUE, "Octree nodes array"=w1533) -> ("Error out"=w1524:errorcluster, "Octree node boxes array"=w1527:refnum<vi>[])
            n364 = Build Array (concatenate)(w1526, w1528, w1527) -> (w1522:refnum<vi>[])
            n365 = Merge Errors(w1525, w1524) -> (w1523:errorcluster)
          }
        }
        n366 = global read "Collision Detection global.vi" "Collision marker radius (mm)"() -> (w1370:sgl)
        n367 = Empty Array?(array=w1343) -> (empty?=w1387:bool)
        n368 = case shown="False" w1387 {
          tunnel: T2 {"Red"=1.0, "Green"=0.0, "Blue"=0.0, "Alpha"=1.0} ("Colour") -> [w1517 _]
          tunnel: w1370 -> [w1516 _]
          tunnel: w1351 -> [w1515 _]
          tunnel: [w1514 errorcluster {"status"=FALSE, "code"=0, "source"=""} ("error IO")] -> w1396
          tunnel: [w1512 w1519] -> w1376
          tunnel: w1377 -> [w1513 w1519]
          tunnel: w1343 -> [w1510 _]
          frame False {
            n369 = call "Create spheres.vi"("Render mode"=w1515, "Colour"=w1517, "Radius (model units)"=w1516, "Points array"=w1510) -> ("Error out"=w1514:errorcluster, "Points"=w1511:refnum<vi>[])
            n370 = Build Array (concatenate)(w1513, w1511) -> (w1512:refnum<vi>[])
          }
          frame True {
          }
        }
        n371 = global read "Collision Detection global.vi" "Camera Position"() -> (w1374:T11)
        n372 = global read "Collision Detection global.vi" "Reset camera"() -> (w1363:bool)
        n373 = global read "Collision Detection global.vi" "Up Direction"() -> (w1372:T11)
        n374 = global read "Collision Detection global.vi" "Target"() -> (w1373:T11)
        n375 = call "Create new scene.vi"("Translation"=cluster{"X":sgl, "Y":sgl, "Z":sgl} {"X"=0.0, "Y"=0.0, "Z"=0.0}, "Scale"=cluster{"X":sgl, "Y":sgl, "Z":sgl} {"X"=1.0, "Y"=1.0, "Z"=1.0}, "Scene objects array"=w1376) -> ("Error out"=w1395:errorcluster, "Scene out"=w1379:refnum<vi>)
        n376 = call "3D display.vi"("Camera Position"=w1374, "Scene in"=w1379, "Target"=w1373, "Up Direction"=w1372, "Reset camera"=w1363) -> ("3D Picture"=w1337:refnum<vi>)
        n377 = Merge Errors(w1394, w1401, w1365, w1350, w1400, w1399, w1398, w1397, w1396, w1395) -> (w1393:errorcluster)
        n378 = Close Reference(reference=w1337) -> ()  [unwired: 1 in, 1 out]
      }
      frame "End" {
        # "Min. sep. dist. is returned as -1 if the option is enabled and no objects were detected within sphere radius.\nNaN is returned if the option is disabled (can use this rather than check the boolean)."
        n379 = case shown="True" w1537 {
          tunnel: w1540 -> [_ w1578]
          tunnel: w1539 -> [_ w1575]
          tunnel: [sgl nan ("t") w1574] -> w1538
          frame False {
          }
          frame True {
            n380 = Empty Array?(array=w1578) -> (empty?=w1577:bool)
            n381 = Select(t=sgl -1.0, s=w1577, f=w1575) -> (s? t:f=w1574:sgl)
          }
        }
        n382 = case shown="True" w1560 {
          tunnel: w1559 -> [_ w1586]
          tunnel: w1558 -> [_ w1585]
          tunnel: w1557 -> [_ w1584]
          tunnel: [w1582 w1586] -> w1556
          tunnel: [w1581 w1585] -> w1555
          tunnel: [w1580 w1584] -> w1554
          tunnel: w1553 -> [w1580 _]
          tunnel: w1552 -> [w1581 _]
          tunnel: w1551 -> [w1582 _]
          tunnel: [w1579 FALSE] -> w1542
          tunnel: w1541 -> [w1579 _]
          frame False {
          }
          frame True {
          }
        }
      }
    }
  }
  "Collision" <- w22
  "Minimum separation" <- w21
  "Minimum separation vector (from trav.)" <- w20
  "Collision point(s)" <- w19
  "Error out" <- w18
  "Traverse collision part" <- w5
